vi "WS1050_Bench_RFFE_Package_FullStep_Multi-VPI_Ver1.4.vi"(4 "Send":bool, 5 "CLICK DOWN TO QUIT":bool=TRUE) -> (0 "EXE SEQ":bool, 1 "POWER ON":bool, 2 "CHARGE \nPUMP ON":bool, 3 "POWER OFF":bool)   [LabVIEW 2017]
uses:
  <instrlib>/Tektronix DPO MSO 2000 4000 Series/Tektronix DPO MSO 2000 4000 Series.lvlib
panel:
  in  "Driver Name":string[](array[string])=["C1_F1_UP", "C1_F1_DN", "C1_F2_UP", "C1_F2_DN", "C1_S1_UP", "C1_S2_UP", "C1_S3_UP", "C1_S4_UP", "C1_S5_UP", "C1_S6_UP", "C1_S7_UP", "C1_S8_UP", "C1_S9_UP", "C1_S10_UP", "C1_S11_UP", "C1_S12_UP", "C1_S13_UP", "C1_S14_UP", "C1_S13_DN", "C1_S12_DN", "C1_S11_DN", "C1_S10_DN", "C1_S9_DN", "C1_S8_DN", "C1_S7_DN", "C1_S6_DN", "C1_S5_DN", "C1_S4_DN", "C1_S3_DN", "C1_S2_DN", "C1_S1_DN", "C1_ALL_DN", "C2_F1_UP", "C2_F1_DN", "C2_F2_UP", "C2_F2_DN", "C2_S1_UP", "C2_S2_UP", "C2_S3_UP", "C2_S4_UP", "C2_S5_UP", "C2_S6_UP", "C2_S7_UP", "C2_S8_UP", "C2_S9_UP", "C2_S10_UP", "C2_S11_UP", "C2_S12_UP", "C2_S13_UP", "C2_S14_UP", "C2_S13_DN", "C2_S12_DN", "C2_S11_DN", "C2_S10_DN", "C2_S9_DN", "C2_S8_DN", "C2_S7_DN", "C2_S6_DN", "C2_S5_DN", "C2_S4_DN", "C2_S3_DN", "C2_S2_DN", "C2_S1_DN", "C2_ALL_DN", "C3_F1_UP", "C3_F1_DN", "C3_F2_UP", "C3_F2_DN", "C3_S1_UP", "C3_S2_UP", "C3_S3_UP", "C3_S4_UP", "C3_S5_UP", "C3_S6_UP", "C3_S7_UP", "C3_S8_UP", "C3_S9_UP", "C3_S10_UP", "C3_S11_UP", "C3_S12_UP", "C3_S13_UP", "C3_S14_UP", "C3_S13_DN", "C3_S12_DN", "C3_S11_DN", "C3_S10_DN", "C3_S9_DN", "C3_S8_DN", "C3_S7_DN", "C3_S6_DN", "C3_S5_DN", "C3_S4_DN", "C3_S3_DN", "C3_S2_DN", "C3_S1_DN", "C3_ALL_DN"]
  out "VPIData Out":string[][](array[string])=[["23.75", "24.688778E+0", "26.641948E+0", "1.143234E+0", "1.456892E+0", "1.305106E+0", "5.842594E+0", "6.189537E+0", "5.965014E+0", "1.144009E+0", "1.457367E+0", "1.305342E+0"], ["25.25", "28.907904E+0", "30.923880E+0", "1.143611E+0", "1.456986E+0", "1.305152E+0", "6.241702E+0", "6.610390E+0", "6.345839E+0", "1.144181E+0", "1.457457E+0", "1.305251E+0"], ["26.75", "29.144374E+0", "31.764876E+0", "1.143694E+0", "1.457180E+0", "1.305124E+0", "6.702805E+0", "7.218784E+0", "6.834179E+0", "1.144211E+0", "1.457512E+0", "1.305239E+0"], ["28.25", "34.886023E+0", "34.072784E+0", "1.143698E+0", "1.457273E+0", "1.305144E+0", "7.038370E+0", "7.580288E+0", "7.141688E+0", "1.144281E+0", "1.457594E+0", "1.305200E+0"], ["29.75", "39.362117E+0", "39.077158E+0", "1.143966E+0", "1.457275E+0", "1.304983E+0", "7.242981E+0", "7.704995E+0", "7.339693E+0", "1.144341E+0", "1.457691E+0", "1.305103E+0"], ["31.25", "42.309906E+0", "40.849836E+0", "1.143915E+0", "1.457288E+0", "1.304925E+0", "7.277188E+0", "7.740502E+0", "7.479733E+0", "1.144306E+0", "1.457570E+0", "1.305177E+0"], ["32.75", "44.234610E+0", "46.055910E+0", "1.143960E+0", "1.457368E+0", "1.305002E+0", "7.280773E+0", "7.734846E+0", "7.488937E+0", "1.144393E+0", "1.457617E+0", "1.305036E+0"], ["36.5", "53.659837E+0", "54.632880E+0", "1.143940E+0", "1.457204E+0", "1.304867E+0", "7.259427E+0", "7.702645E+0", "7.475886E+0", "1.144397E+0", "1.457589E+0", "1.304969E+0"], ["38", "59.644864E+0", "60.152367E+0", "1.143951E+0", "1.457364E+0", "1.304848E+0", "7.261446E+0", "7.706233E+0", "7.483841E+0", "1.144378E+0", "1.457810E+0", "1.304931E+0"], ["39.5", "63.989183E+0", "65.317284E+0", "1.143941E+0", "1.457225E+0", "1.304758E+0", "7.265702E+0", "7.716856E+0", "7.496982E+0", "1.144459E+0", "1.457567E+0", "1.305018E+0"], ["41", "71.621806E+0", "72.420343E+0", "1.143974E+0", "1.457385E+0", "1.304771E+0", "7.280796E+0", "7.729684E+0", "7.509736E+0", "1.144398E+0", "1.457685E+0", "1.304964E+0"], ["42.5", "79.427320E+0", "78.815208E+0", "1.144006E+0", "1.457337E+0", "1.304647E+0", "7.294107E+0", "7.742713E+0", "7.524602E+0", "1.144470E+0", "1.457591E+0", "1.304984E+0"], ["50", "124.732767E+0", "124.448999E+0", "1.143917E+0", "1.457358E+0", "1.304779E+0", "7.355203E+0", "7.811398E+0", "7.595755E+0", "1.144361E+0", "1.457583E+0", "1.304904E+0"]]
  in  "Sequence Names_Test":string[](array[string])=["CMin_VPI", "C1_VPI", "C2_VPI", "C3_VPI", "ALL_ON_VPI", "ALL_OFF_VPI"]
  out "Bank C1":string[](array[string])=["1.263962E+0", "1.365449E+0", "1.485278E+0", "1.432169E+0", "1.551803E+0", "1.653654E+0", "1.773449E+0", "1.874928E+0", "1.994661E+0", "2.096378E+0", "2.216085E+0", "2.295742E+0", "2.415533E+0", "2.517390E+0", "2.637083E+0", "2.682913E+0", "2.802580E+0", "2.904045E+0", "3.023833E+0", "3.131829E+0", "3.251440E+0", "3.353096E+0", "3.472585E+0", "3.523851E+0", "3.643284E+0", "3.745093E+0", "3.864497E+0", "3.961956E+0", "4.081577E+0", "4.183076E+0", "4.302464E+0", "4.402392E+0", "4.521881E+0", "4.623312E+0", "4.742844E+0", "4.829751E+0", "4.949292E+0", "5.050642E+0", "5.170100E+0", "5.220759E+0", "5.340368E+0", "5.441944E+0", "5.561578E+0", "5.635534E+0", "5.754912E+0", "5.856368E+0", "5.975750E+0", "6.045793E+0", "6.165061E+0", "6.266516E+0", "6.385998E+0", "6.487936E+0", "6.607210E+0", "6.708605E+0", "6.827699E+0", "6.897334E+0", "7.016852E+0", "7.117872E+0", "7.237418E+0", "7.119044E+0", "7.017414E+0", "6.898357E+0", "6.828583E+0", "6.709397E+0", "6.608499E+0", "6.489420E+0", "6.387433E+0", "6.268261E+0", "6.167466E+0", "6.048157E+0", "5.978147E+0", "5.859144E+0", "5.757853E+0", "5.638742E+0", "5.564712E+0", "5.445596E+0", "5.344232E+0", "5.225011E+0", "5.172354E+0", "5.053104E+0", "4.951765E+0", "4.832427E+0", "4.745420E+0", "4.626077E+0", "4.524684E+0", "4.405379E+0", "4.305223E+0", "4.185939E+0", "4.084376E+0", "3.964977E+0", "3.867230E+0", "3.747748E+0", "3.646212E+0", "3.526797E+0", "3.475012E+0", "3.355543E+0", "3.253861E+0", "3.134287E+0", "3.026013E+0", "2.906604E+0", "2.804812E+0", "2.685213E+0", "2.639527E+0", "2.519887E+0", "2.418143E+0", "2.298505E+0", "2.217875E+0", "2.098228E+0", "1.996638E+0", "1.876815E+0", "1.775184E+0", "1.655537E+0", "1.553577E+0", "1.433939E+0", "1.486023E+0", "1.366138E+0", "1.264338E+0", "1.144571E+0"]
  in  "Cmd Full":string[](array[string])=["01", "02", "03", "04", "05", "06", "07", "08", "09", "0A", "0B", "0C", "0D", "0E", "0F", "10", "11", "12", "13", "14", "15", "16", "17", "18", "19", "1A", "1B", "1C", "1D", "1E", "1F", "20", "21", "22", "23", "24", "25", "26", "27", "28", "29", "2A", "2B", "2C", "2D", "2E", "2F", "30", "31", "32", "33", "34", "35", "36", "37", "38", "39", "3A", "3B", "3A", "39", "38", "37", "36", "35", "34", "33", "32", "31", "30", "2F", "2E", "2D", "2C", "2B", "2A", "29", "28", "27", "26", "25", "24", "23", "22", "21", "20", "1F", "1E", "1D", "1C", "1B", "1A", "19", "18", "17", "16", "15", "14", "13", "12", "11", "10", "0F", "0E", "0D", "0C", "0B", "0A", "09", "08", "07", "06", "05", "04", "03", "02", "01", "00"]
  in  "Driver Name Full":string[](array[string])=["S0F1_UP", "S0F2_UP", "S0F12_UP", "S1_UP", "S1F1_UP", "S1F2_UP", "S1F12_UP", "S2_UP", "S2F1_UP", "S2F2_UP", "S2F12_UP", "S3_UP", "S3F1_UP", "S3F2_UP", "S3F12_UP", "S4_UP", "S4F1_UP", "S4F2_UP", "S4F12_UP", "S5_UP", "S5F1_UP", "S5F2_UP", "S5F12_UP", "S6_UP", "S6F1_UP", "S6F2_UP", "S6F12_UP", "S7_UP", "S7F1_UP", "S7F2_UP", "S7F12_UP", "S8_UP", "S8F1_UP", "S8F2_UP", "S8F12_UP", "S9_UP", "S9F1_UP", "S9F2_UP", "S9F12_UP", "S10_UP", "S10F1_UP", "S10F2_UP", "S10F12_UP", "S11_UP", "S11F1_UP", "S11F2_UP", "S11F12_UP", "S12_UP", "S12F1_UP", "S12F2_UP", "S12F12_UP", "S13_UP", "S13F1_UP", "S13F2_UP", "S13F12_UP", "S14_UP", "S14F1_UP", "S14F2_UP", "S14F12_UP", "S14F2_DN", "S14F1_DN", "S14_DN", "S13F12_DN", "S13F2_DN", "S13F1_DN", "S13_DN", "S12F12_DN", "S12F2_DN", "S12F1_DN", "S12_DN", "S11F12_DN", "S11F2_DN", "S11F1_DN", "S11_DN", "S10F12_DN", "S10F2_DN", "S10F1_DN", "S10_DN", "S9F12_DN", "S9F2_DN", "S9F1_DN", "S9_DN", "S8F12_DN", "S8F2_DN", "S8F1_DN", "S8_DN", "S7F12_DN", "S7F2_DN", "S7F1_DN", "S7_DN", "S6F12_DN", "S6F2_DN", "S6F1_DN", "S6_DN", "S5F12_DN", "S5F2_DN", "S5F1_DN", "S5_DN", "S4F12_DN", "S4F2_DN", "S4F1_DN", "S4_DN", "S3F12_DN", "S3F2_DN", "S3F1_DN", "S3_DN", "S2F12_DN", "S2F2_DN", "S2F1_DN", "S2_DN", "S1F12_DN", "S1F2_DN", "S1F1_DN", "S1_DN", "S0F12_DN", "S0F2_DN", "S0F1_DN", "ALL_OFF"]
  in  "WS1050 C3L Cmd":string[](array[string])=["074301", "074300", "074302", "074300", "074304", "074308", "07430C", "074310", "074314", "074318", "07431C", "074320", "074324", "074328", "07432C", "074330", "074334", "074338", "074339", "07433B", "074339", "074338", "074334", "074330", "07432C", "074328", "074324", "074320", "07431C", "074318", "074314", "074310", "07430C", "074308", "074304", "074300"]
  in  "C3L":string[](array[string])=["C3L_S0F1_ON", "C3L_S0F1_OFF", "C3L_S0F2_ON", "C3L_S0F2_OFF", "C3L_S1_UP", "C3L_S2_UP", "C3L_S3_UP", "C3L_S4_UP", "C3L_S5_UP", "C3L_S6_UP", "C3L_S7_UP", "C3L_S8_UP", "C3L_S9_UP", "C3L_S10_UP", "C3L_S11_UP", "C3L_S12_UP", "C3L_S13_UP", "C3L_S14_UP", "C3L_S14F1_UP", "C3L_S14F12_UP", "C3L_S14F1_DN", "C3L_S14_DN", "C3L_S13_DN", "C3L_S12_DN", "C3L_S11_DN", "C3L_S10_DN", "C3L_S9_DN", "C3L_S8_DN", "C3L_S7_DN", "C3L_S6_DN", "C3L_S5_DN", "C3L_S4_DN", "C3L_S3_DN", "C3L_S2_DN", "C3L_S1_DN", "C3L_ALL_OFF"]
  in  "WS1050 C2L Cmd":string[](array[string])=["074201", "074200", "074202", "074200", "074204", "074208", "07420C", "074210", "074214", "074218", "07421C", "074220", "074224", "074228", "07422C", "074230", "074234", "074238", "074239", "07423B", "074239", "074238", "074234", "074230", "07422C", "074228", "074224", "074220", "07421C", "074218", "074214", "074210", "07420C", "074208", "074204", "074200"]
  in  "C2L":string[](array[string])=["C2L_S0F1_ON", "C2L_S0F1_OFF", "C2L_S0F2_ON", "C2L_S0F2_OFF", "C2L_S1_UP", "C2L_S2_UP", "C2L_S3_UP", "C2L_S4_UP", "C2L_S5_UP", "C2L_S6_UP", "C2L_S7_UP", "C2L_S8_UP", "C2L_S9_UP", "C2L_S10_UP", "C2L_S11_UP", "C2L_S12_UP", "C2L_S13_UP", "C2L_S14_UP", "C2L_S14F1_UP", "C2L_S14F12_UP", "C2L_S14F1_DN", "C2L_S14_DN", "C2L_S13_DN", "C2L_S12_DN", "C2L_S11_DN", "C2L_S10_DN", "C2L_S9_DN", "C2L_S8_DN", "C2L_S7_DN", "C2L_S6_DN", "C2L_S5_DN", "C2L_S4_DN", "C2L_S3_DN", "C2L_S2_DN", "C2L_S1_DN", "C2L_ALL_OFF"]
  in  "C1 Cmd":string[](array[string])=["074101", "074100", "074102", "074100", "074104", "074108", "07410C", "074110", "074114", "074118", "07411C", "074120", "074124", "074128", "07412C", "074130", "074134", "074138", "074139", "07413B", "074139", "074138", "074134", "074130", "07412C", "074128", "074124", "074120", "07411C", "074118", "074114", "074110", "07410C", "074108", "074104", "074100"]
  in  "C1":string[](array[string])=["C1L_S0F1_ON", "C1L_S0F1_OFF", "C1L_S0F2_ON", "C1L_S0F2_OFF", "C1L_S1_UP", "C1L_S2_UP", "C1L_S3_UP", "C1L_S4_UP", "C1L_S5_UP", "C1L_S6_UP", "C1L_S7_UP", "C1L_S8_UP", "C1L_S9_UP", "C1L_S10_UP", "C1L_S11_UP", "C1L_S12_UP", "C1L_S13_UP", "C1L_S14_UP", "C1L_S14F1_UP", "C1L_S14F12_UP", "C1L_S14F1_DN", "C1L_S14_DN", "C1L_S13_DN", "C1L_S12_DN", "C1L_S11_DN", "C1L_S10_DN", "C1L_S9_DN", "C1L_S8_DN", "C1L_S7_DN", "C1L_S6_DN", "C1L_S5_DN", "C1L_S4_DN", "C1L_S3_DN", "C1L_S2_DN", "C1L_S1_DN", "C1L_ALL_OFF"]
  out "CMin Delay_AST":string[](array[string])=["0.000000E+0", "1.143716E+0", "1.458036E+0", "1.306985E+0", "0.000000E+0", "1.143733E+0", "1.457970E+0", "1.306825E+0", "0.000000E+0", "1.143759E+0", "1.458098E+0", "1.306746E+0", "0.000000E+0", "1.143710E+0", "1.457896E+0", "1.306740E+0"]
  in  "Reg1_Bit Cntrl 2":string[](array[string])=["01", "02", "04", "08", "10", "20", "40", "80", "03", "06", "0C", "D8", "33", "66", "CC", "07", "0E", "1C", "38", "70", "E0", "0F", "1E", "3C", "78", "F0", "1F", "3E", "7C", "F8", "3F", "7E", "FC", "7F", "FE", "FD", "FB", "F7", "EF", "DF", "BF", "7F", "FC", "F9", "F3", "E7", "CF", "9F", "3F", "F8", "F1", "E3", "C7", "8F", "1F", "F0", "E1", "C3", "87", "0F", "E0", "C1", "83", "07", "C0", "81", "03", "AA", "55", "00"]
  out "CMin C3(pF)":dbl=1.3051738281250005
  out "Delta_C3(pF)":dbl=6.016130171874999
  out "CMin C2(pF)":dbl=1.4578437500000003
  out "Delta_C2(pF)":dbl=6.2455592499999995
  out "Delta_C1(pF)":dbl=6.0930322578125
  out "CMin C1(pF)":dbl=1.1443857421874997
  in  "Tab Control":T1(tab)=enum."Indicator"
  in  "Select CPV":i32(ring)=1 items=["CP_35V", "CP_40.25V", "CP_41V", "CP_42.5V", "CP_44V", "CP_50V", "CP_55V"]
  in  "Header Table":string[][](table)=[["Lot#", "Wafer#", "SN#", "", "", "", "", "", "I_total"], ["WS1050", "T7", "1", "", "", "", "", "", "0.000000E+0"]]
  in  "TMN DC\\CAP Data Log File Path":path=path "C:/Andy/WS1050/Full TP/Multi VPI"
  out "2K Cycles":bool
  out "Pass /Fail?":bool=TRUE
  in  "Config File Path":path=path "S:/Software_Control/RELEASED_SOFTWARE_RUN_ALL_TEST_FROM_HERE/PACKAGE/TMN/TMN1P5-Test-System/WS1050_vsa20-20_Temp.txt"
  in  "Title":string="WS1050_Bench_RFFE_Package_Full_Multi-VPI Ver1.4"
  in  "Allowed (pF)":dbl=1.9898
  out "Difference":dbl=0.04109082031250022
  out "IDD_Stdby":string="652.477375E-3"
  out "C2Cal (pF)":dbl=-4.9191376953125
  out "C1Cal (pF)":dbl=-4.5642919921875
  out "C3Cal (pF)":dbl=-4.9974111328125
  in  "Bench #":string="1A"
  in  "Init AD7747":bool
  out "% Delta Cap":dbl=82.95919403248587 format="%#_5g"
  in  "VDD \nSet Up":dbl=3.3 format="%.2p"
  out "C2":dbl=1.4562451171874997
  out "C3":dbl=1.3041181640625004
  out "C1":dbl=1.1432705078124998
  in  "S-Time":bool=TRUE
  in  "GROUP":string
  out "HS \nCheck":bool=TRUE
  in  "Delay Cap Meas":u32=100
  out "Sequence":i32(listbox)=5
  out "IDD_All ON":string="36.261307E+0"
  out "IDD_All OFF":string="34.905880E+0"
  in  "Scope Set Up":bool
  in  "Manual CP Setting":i32(ring) items=["CP OFF", "CP ON", "DVA OFF", "DVA ON", "ECAL OFF", "ECAL ON", "CP 40.25V", "CP 35V", "CP 38V", "CP 44V", "CP 50V", "CP 23.75V", "CP 25.25V", "CP 29.75V", "C1 ON", "C1 OFF", "C2 ON", "C2 OFF", "C3 ON", "C3 OFF"]
  out "Bins":string="111111111"
  in  "Calib\nSocket":bool
  in  "BurnIn Efuse":bool
  out "S_ValueC2(pF)":dbl=-4.9191376953125
  out "S_ValueC1(pF)":dbl=-4.5642919921875
  out "S_ValueC3(pF)":dbl=-4.9974111328125
  out "Status":string="Idle....."
  in  "CMOS Setup":T2={"ECAL"=FALSE, "Full Steps"=TRUE, "Multi VPI"=TRUE, "DVA"=FALSE, "EFuse RB"=TRUE, "Init RB"=TRUE, "HS Test"=TRUE}
  in  "Comment":string="Init Run"
  out "IDD_VPI ON":string="124.448999E+0"
  out "IDD_VPI OFF":string="43.360206E+0"
  in  "Delta C Target":dbl=22.125
  in  "IDD Limit":dbl=0.02 format="%.2p"
  out "CMOS Out":T3
  out "Pass/Fail":bool
  in  "START \nTEST":bool
  in  "Save/Recal":u16(ring)=1 items=["Save", "Recall"]
  in  "Location":u16(ring)=1 items=["Location 1"=1, "Location 2"=2, "Location 3"=3, "Location 4"=4, "Location 5"=5, "Location 6"=6, "Location 7"=7, "Location 8"=8, "Location 9"=9, "Location 10"=10]
  in  "Dev 6501":tag="Dev2/port2/line0" caption="Lines"
  in  "Ke2400_VSA":refnum<visa-resource-name>="GPIB1::1::INSTR"
  in  "Scope USB":refnum<visa-resource-name>="USB0::0x0699::0x0405::C010240::INSTR"
  in  "Ke2000_IDD":refnum<visa-resource-name>="GPIB1::9::INSTR"
  in  "A364X_VDD":refnum<visa-resource-name>="GPIB1::6::INSTR"
  in  "RFFE":refnum<visa-resource-name>="COM3"
  in  "CAP Meas":refnum<visa-resource-name>="COM8"
  in  "% Amp_T2":dbl=0.9
  in  "% Amp_T1":dbl=0.6
  in  "% Amp_T3":dbl=0.95
  out "C1 Graph":dbl[](graph)=[0.0, 1.263962, 1.365449, 1.485278, 1.432169, 1.551803, 1.653654, 1.773449, 1.874928, 1.994661, 2.096378, 2.216085, 2.295742, 2.415533, 2.51739, 2.637083, 2.682913, 2.80258, 2.904045, 3.023833, 3.131829, 3.25144, 3.353096, 3.472585, 3.523851, 3.643284, 3.745093, 3.864497, 3.961956, 4.081577, 4.183076, 4.302464, 4.402392, 4.521881, 4.623312, 4.742844, 4.829751, 4.949292, 5.050642, 5.1701, 5.220759, 5.340368, 5.441944, 5.561578, 5.635534, 5.754912, 5.856368, 5.97575, 6.045793, 6.165061, 6.266516, 6.385998, 6.487936, 6.60721, 6.708605, 6.827699, 6.897334, 7.016852, 7.117872, 7.237418, 7.119044, 7.017414, 6.898357, 6.828583, 6.709397, 6.608499, 6.48942, 6.387433, 6.268261, 6.167466, 6.048157, 5.978147, 5.859144, 5.757853, 5.638742, 5.564712, 5.445596, 5.344232, 5.225011, 5.172354, 5.053104, 4.951765, 4.832427, 4.74542, 4.626077, 4.524684, 4.405379, 4.305223, 4.185939, 4.084376, 3.964977, 3.86723, 3.747748, 3.646212, 3.526797, 3.475012, 3.355543, 3.253861, 3.134287, 3.026013, 2.906604, 2.804812, 2.685213, 2.639527, 2.519887, 2.418143, 2.298505, 2.217875, 2.098228, 1.996638, 1.876815, 1.775184, 1.655537, 1.553577, 1.433939, 1.486023, 1.366138, 1.264338, 1.144571]
  out "C3 Graph":dbl[](graph)=[0.0, 1.422279, 1.529396, 1.647592, 1.587427, 1.705936, 1.813056, 1.931501, 2.010594, 2.12888, 2.236136, 2.354354, 2.442663, 2.560794, 2.668117, 2.786146, 2.836266, 2.954609, 3.061958, 3.180341, 3.261733, 3.37968, 3.48677, 3.605037, 3.668454, 3.787129, 3.894527, 4.012835, 4.070176, 4.188148, 4.295722, 4.413869, 4.460793, 4.579203, 4.686998, 4.804826, 4.863056, 4.981473, 5.088459, 5.206437, 5.295951, 5.414221, 5.521045, 5.638942, 5.718083, 5.835798, 5.942316, 6.060159, 6.166447, 6.284119, 6.391635, 6.509771, 6.557677, 6.675995, 6.782858, 6.900237, 6.978327, 7.095955, 7.202923, 7.321304, 7.203739, 7.097227, 6.979802, 6.901916, 6.784847, 6.678636, 6.561449, 6.514128, 6.396538, 6.289368, 6.171697, 6.065714, 5.948443, 5.841961, 5.725111, 5.645481, 5.528093, 5.421427, 5.303914, 5.214352, 5.097081, 4.990326, 4.87318, 4.814867, 4.69695, 4.590414, 4.473239, 4.422443, 4.3051, 4.197548, 4.08006, 4.021558, 3.903968, 3.797943, 3.679766, 3.609854, 3.491904, 3.384882, 3.266992, 3.185201, 3.067382, 2.960379, 2.842307, 2.791841, 2.673946, 2.566588, 2.448998, 2.359516, 2.241886, 2.135073, 2.016561, 1.936616, 1.818586, 1.711329, 1.593368, 1.648649, 1.53052, 1.423407, 1.305246]
  out "C2 Graph":dbl[](graph)=[0.0, 1.585713, 1.689148, 1.817662, 1.885455, 2.014188, 2.117619, 2.24629, 2.237105, 2.36588, 2.469066, 2.597716, 2.654179, 2.782699, 2.886215, 3.01476, 3.089162, 3.217774, 3.321294, 3.449749, 3.491522, 3.620192, 3.723275, 3.851945, 3.887914, 4.016458, 4.119716, 4.248221, 4.339437, 4.467828, 4.570915, 4.6994, 4.71226, 4.840867, 4.944326, 5.072629, 5.17246, 5.301332, 5.404473, 5.532792, 5.631586, 5.759431, 5.862757, 5.990751, 6.053234, 6.181604, 6.284377, 6.412689, 6.511694, 6.639869, 6.743027, 6.87107, 6.936174, 7.064378, 7.167445, 7.295804, 7.344181, 7.472198, 7.575125, 7.703403, 7.57569, 7.472819, 7.345312, 7.296507, 7.168775, 7.06663, 6.93829, 6.872623, 6.744731, 6.642141, 6.513973, 6.41498, 6.28691, 6.183715, 6.055874, 5.993849, 5.86599, 5.762587, 5.63454, 5.535872, 5.407794, 5.304726, 5.176538, 5.076043, 4.947812, 4.845088, 4.716747, 4.702071, 4.573709, 4.470539, 4.342157, 4.250793, 4.122445, 4.019188, 3.890785, 3.854401, 3.725925, 3.622958, 3.494537, 3.452021, 3.323469, 3.220432, 3.091716, 3.016233, 2.887631, 2.784359, 2.655705, 2.598903, 2.470368, 2.36705, 2.23842, 2.247739, 2.119168, 2.01572, 1.887002, 1.81881, 1.690278, 1.586776, 1.45797]
  out "Init EFuse RB":string[](array[string])=["40", "00", "00", "00", "28", "50", "00", "F3", "00", "00"]
  out "EFuse 1":string="50"
  out "EFuse 2":string="50"
  out "EUSE Burn":string[](array[string])=["n/a", "n/a"]
  out "I_stdby End":string="99.571387E+0"
  out "RB All Regs Dump":string[](array[string])=["44", "3B", "3B", "3B", "28", "50", "00", "F3", "00", "00", "44", "00", "00", "00", "28", "50", "00", "F3", "00", "00", "44", "00", "00", "00", "28", "50", "00", "EF", "20", "00", "44", "3B", "3B", "3B", "28", "50", "00", "EF", "20", "00", "44", "00", "00", "00", "28", "50", "00", "FB", "20", "00", "44", "3B", "3B", "3B", "28", "50", "00", "FB", "20", "00", "44", "00", "00", "00", "28", "50", "00", "F6", "20", "00", "44", "3B", "3B", "3B", "28", "50", "00", "F6", "20", "00"]
  in  "RB All Regs":bool=TRUE
  in  "CMin Delay":string[](array[string])=["0", "0", "0", "0"]
  in  "CMin/Delay":bool
  out "Ke2400 out":refnum<visa-resource-name>
  out "VDD Out Dup":refnum<visa-resource-name>
  out "Error Out":errorcluster
  out "AST":errorcluster
  out "Completed":errorcluster
  out "RFFE Out After Test":errorcluster
  out "Signal":dbl[](graph)
  out "Filtered Signal":dbl[](graph)
  out "After RB":errorcluster
  out "Power OFF":errorcluster
  out "Lot":string="WS1050"
  out "Wafer":string="T7"
  out "All Out":string[](array[string])=["4/7/2014", "4:26:21 PM", "WS1050", "T7", "1", "40", "00", "00", "00", "28", "50", "00", "F3", "00", "00", "Pass", "50", "50", "652.477375E-3", "34.905880E+0", "36.261307E+0", "1.144386E+0", "1.457844E+0", "1.305174E+0", "1.263962E+0", "1.365449E+0", "1.485278E+0", "1.432169E+0", "1.551803E+0", "1.653654E+0", "1.773449E+0", "1.874928E+0", "1.994661E+0", "2.096378E+0", "2.216085E+0", "2.295742E+0", "2.415533E+0", "2.517390E+0", "2.637083E+0", "2.682913E+0", "2.802580E+0", "2.904045E+0", "3.023833E+0", "3.131829E+0", "3.251440E+0", "3.353096E+0", "3.472585E+0", "3.523851E+0", "3.643284E+0", "3.745093E+0", "3.864497E+0", "3.961956E+0", "4.081577E+0", "4.183076E+0", "4.302464E+0", "4.402392E+0", "4.521881E+0", "4.623312E+0", "4.742844E+0", "4.829751E+0", "4.949292E+0", "5.050642E+0", "5.170100E+0", "5.220759E+0", "5.340368E+0", "5.441944E+0", "5.561578E+0", "5.635534E+0", "5.754912E+0", "5.856368E+0", "5.975750E+0", "6.045793E+0", "6.165061E+0", "6.266516E+0", "6.385998E+0", "6.487936E+0", "6.607210E+0", "6.708605E+0", "6.827699E+0", "6.897334E+0", "7.016852E+0", "7.117872E+0", "7.237418E+0", "7.119044E+0", "7.017414E+0", "6.898357E+0", "6.828583E+0", "6.709397E+0", "6.608499E+0", "6.489420E+0", "6.387433E+0", "6.268261E+0", "6.167466E+0", "6.048157E+0", "5.978147E+0", "5.859144E+0", "5.757853E+0", "5.638742E+0", "5.564712E+0", "5.445596E+0", "5.344232E+0", "5.225011E+0", "5.172354E+0", "5.053104E+0", "4.951765E+0", "4.832427E+0", "4.745420E+0", "4.626077E+0", "4.524684E+0", "4.405379E+0", "4.305223E+0", "4.185939E+0", "4.084376E+0", "3.964977E+0", "3.867230E+0", "3.747748E+0", "3.646212E+0", "3.526797E+0", "3.475012E+0", "3.355543E+0", "3.253861E+0", "3.134287E+0", "3.026013E+0", "2.906604E+0", "2.804812E+0", "2.685213E+0", "2.639527E+0", "2.519887E+0", "2.418143E+0", "2.298505E+0", "2.217875E+0", "2.098228E+0", "1.996638E+0", "1.876815E+0", "1.775184E+0", "1.655537E+0", "1.553577E+0", "1.433939E+0", "1.486023E+0", "1.366138E+0", "1.264338E+0", "1.144571E+0", "1.195763E-1", "2.210633E-1", "3.408923E-1", "2.877833E-1", "4.074173E-1", "5.092683E-1", "6.290633E-1", "7.305423E-1", "8.502753E-1", "9.519923E-1", "1.071699E+0", "1.151356E+0", "1.271147E+0", "1.373004E+0", "1.492697E+0", "1.538527E+0", "1.658194E+0", "1.759659E+0", "1.879447E+0", "1.987443E+0", "2.107054E+0", "2.208710E+0", "2.328199E+0", "2.379465E+0", "2.498898E+0", "2.600707E+0", "2.720111E+0", "2.817570E+0", "2.937191E+0", "3.038690E+0", "3.158078E+0", "3.258006E+0", "3.377495E+0", "3.478926E+0", "3.598458E+0", "3.685365E+0", "3.804906E+0", "3.906256E+0", "4.025714E+0", "4.076373E+0", "4.195982E+0", "4.297558E+0", "4.417192E+0", "4.491148E+0", "4.610526E+0", "4.711982E+0", "4.831364E+0", "4.901407E+0", "5.020675E+0", "5.122130E+0", "5.241612E+0", "5.343550E+0", "5.462824E+0", "5.564219E+0", "5.683313E+0", "5.752948E+0", "5.872466E+0", "5.973486E+0", "3.760000E-4", "6.890000E-4", "7.450000E-4", "1.770000E-3", "1.774000E-3", "1.883000E-3", "1.735000E-3", "1.887000E-3", "1.977000E-3", "1.850000E-3", "1.790000E-3", "2.763000E-3", "2.610000E-3", "2.497000E-3", "2.444000E-3", "2.300000E-3", "2.232000E-3", "2.559000E-3", "2.180000E-3", "2.458000E-3", "2.421000E-3", "2.447000E-3", "2.427000E-3", "2.946000E-3", "2.928000E-3", "2.655000E-3", "2.733000E-3", "3.021000E-3", "2.799000E-3", "2.863000E-3", "2.759000E-3", "2.987000E-3", "2.803000E-3", "2.765000E-3", "2.576000E-3", "2.676000E-3", "2.473000E-3", "2.462000E-3", "2.254000E-3", "4.252000E-3", "3.864000E-3", "3.652000E-3", "3.134000E-3", "3.208000E-3", "2.941000E-3", "2.776000E-3", "2.397000E-3", "2.364000E-3", "2.405000E-3", "1.745000E-3", "1.435000E-3", "1.484000E-3", "1.289000E-3", "7.920000E-4", "8.840000E-4", "1.023000E-3", "5.620000E-4", "1.172000E-3", "1.585713E+0", "1.689148E+0", "1.817662E+0", "1.885455E+0", "2.014188E+0", "2.117619E+0", "2.246290E+0", "2.237105E+0", "2.365880E+0", "2.469066E+0", "2.597716E+0", "2.654179E+0", "2.782699E+0", "2.886215E+0", "3.014760E+0", "3.089162E+0", "3.217774E+0", "3.321294E+0", "3.449749E+0", "3.491522E+0", "3.620192E+0", "3.723275E+0", "3.851945E+0", "3.887914E+0", "4.016458E+0", "4.119716E+0", "4.248221E+0", "4.339437E+0", "4.467828E+0", "4.570915E+0", "4.699400E+0", "4.712260E+0", "4.840867E+0", "4.944326E+0", "5.072629E+0", "5.172460E+0", "5.301332E+0", "5.404473E+0", "5.532792E+0", "5.631586E+0", "5.759431E+0", "5.862757E+0", "5.990751E+0", "6.053234E+0", "6.181604E+0", "6.284377E+0", "6.412689E+0", "6.511694E+0", "6.639869E+0", "6.743027E+0", "6.871070E+0", "6.936174E+0", "7.064378E+0", "7.167445E+0", "7.295804E+0", "7.344181E+0", "7.472198E+0", "7.575125E+0", "7.703403E+0", "7.575690E+0", "7.472819E+0", "7.345312E+0", "7.296507E+0", "7.168775E+0", "7.066630E+0", "6.938290E+0", "6.872623E+0", "6.744731E+0", "6.642141E+0", "6.513973E+0", "6.414980E+0", "6.286910E+0", "6.183715E+0", "6.055874E+0", "5.993849E+0", "5.865990E+0", "5.762587E+0", "5.634540E+0", "5.535872E+0", "5.407794E+0", "5.304726E+0", "5.176538E+0", "5.076043E+0", "4.947812E+0", "4.845088E+0", "4.716747E+0", "4.702071E+0", "4.573709E+0", "4.470539E+0", "4.342157E+0", "4.250793E+0", "4.122445E+0", "4.019188E+0", "3.890785E+0", "3.854401E+0", "3.725925E+0", "3.622958E+0", "3.494537E+0", "3.452021E+0", "3.323469E+0", "3.220432E+0", "3.091716E+0", "3.016233E+0", "2.887631E+0", "2.784359E+0", "2.655705E+0", "2.598903E+0", "2.470368E+0", "2.367050E+0", "2.238420E+0", "2.247739E+0", "2.119168E+0", "2.015720E+0", "1.887002E+0", "1.818810E+0", "1.690278E+0", "1.586776E+0", "1.457970E+0", "1.278692E-1", "2.313042E-1", "3.598182E-1", "4.276112E-1", "5.563442E-1", "6.597752E-1", "7.884462E-1", "7.792612E-1", "9.080362E-1", "1.011222E+0", "1.139872E+0", "1.196335E+0", "1.324855E+0", "1.428371E+0", "1.556916E+0", "1.631318E+0", "1.759930E+0", "1.863450E+0", "1.991905E+0", "2.033678E+0", "2.162348E+0", "2.265431E+0", "2.394101E+0", "2.430070E+0", "2.558614E+0", "2.661872E+0", "2.790377E+0", "2.881593E+0", "3.009984E+0", "3.113071E+0", "3.241556E+0", "3.254416E+0", "3.383023E+0", "3.486482E+0", "3.614785E+0", "3.714616E+0", "3.843488E+0", "3.946629E+0", "4.074948E+0", "4.173742E+0", "4.301587E+0", "4.404913E+0", "4.532907E+0", "4.595390E+0", "4.723760E+0", "4.826533E+0", "4.954845E+0", "5.053850E+0", "5.182025E+0", "5.285183E+0", "5.413226E+0", "5.478330E+0", "5.606534E+0", "5.709601E+0", "5.837960E+0", "5.886337E+0", "6.014354E+0", "6.117281E+0", "1.063000E-3", "1.130000E-3", "1.148000E-3", "1.547000E-3", "1.532000E-3", "1.549000E-3", "1.449000E-3", "1.315000E-3", "1.170000E-3", "1.302000E-3", "1.187000E-3", "1.526000E-3", "1.660000E-3", "1.416000E-3", "1.473000E-3", "2.554000E-3", "2.658000E-3", "2.175000E-3", "2.272000E-3", "3.015000E-3", "2.766000E-3", "2.650000E-3", "2.456000E-3", "2.871000E-3", "2.730000E-3", "2.729000E-3", "2.572000E-3", "2.720000E-3", "2.711000E-3", "2.794000E-3", "2.671000E-3", "4.487000E-3", "4.221000E-3", "3.486000E-3", "3.414000E-3", "4.078000E-3", "3.394000E-3", "3.321000E-3", "3.080000E-3", "2.954000E-3", "3.156000E-3", "3.233000E-3", "3.098000E-3", "2.640000E-3", "2.111000E-3", "2.533000E-3", "2.291000E-3", "2.279000E-3", "2.272000E-3", "1.704000E-3", "1.553000E-3", "2.116000E-3", "2.252000E-3", "1.330000E-3", "7.030000E-4", "1.131000E-3", "6.210000E-4", "5.650000E-4", "1.422279E+0", "1.529396E+0", "1.647592E+0", "1.587427E+0", "1.705936E+0", "1.813056E+0", "1.931501E+0", "2.010594E+0", "2.128880E+0", "2.236136E+0", "2.354354E+0", "2.442663E+0", "2.560794E+0", "2.668117E+0", "2.786146E+0", "2.836266E+0", "2.954609E+0", "3.061958E+0", "3.180341E+0", "3.261733E+0", "3.379680E+0", "3.486770E+0", "3.605037E+0", "3.668454E+0", "3.787129E+0", "3.894527E+0", "4.012835E+0", "4.070176E+0", "4.188148E+0", "4.295722E+0", "4.413869E+0", "4.460793E+0", "4.579203E+0", "4.686998E+0", "4.804826E+0", "4.863056E+0", "4.981473E+0", "5.088459E+0", "5.206437E+0", "5.295951E+0", "5.414221E+0", "5.521045E+0", "5.638942E+0", "5.718083E+0", "5.835798E+0", "5.942316E+0", "6.060159E+0", "6.166447E+0", "6.284119E+0", "6.391635E+0", "6.509771E+0", "6.557677E+0", "6.675995E+0", "6.782858E+0", "6.900237E+0", "6.978327E+0", "7.095955E+0", "7.202923E+0", "7.321304E+0", "7.203739E+0", "7.097227E+0", "6.979802E+0", "6.901916E+0", "6.784847E+0", "6.678636E+0", "6.561449E+0", "6.514128E+0", "6.396538E+0", "6.289368E+0", "6.171697E+0", "6.065714E+0", "5.948443E+0", "5.841961E+0", "5.725111E+0", "5.645481E+0", "5.528093E+0", "5.421427E+0", "5.303914E+0", "5.214352E+0", "5.097081E+0", "4.990326E+0", "4.873180E+0", "4.814867E+0", "4.696950E+0", "4.590414E+0", "4.473239E+0", "4.422443E+0", "4.305100E+0", "4.197548E+0", "4.080060E+0", "4.021558E+0", "3.903968E+0", "3.797943E+0", "3.679766E+0", "3.609854E+0", "3.491904E+0", "3.384882E+0", "3.266992E+0", "3.185201E+0", "3.067382E+0", "2.960379E+0", "2.842307E+0", "2.791841E+0", "2.673946E+0", "2.566588E+0", "2.448998E+0", "2.359516E+0", "2.241886E+0", "2.135073E+0", "2.016561E+0", "1.936616E+0", "1.818586E+0", "1.711329E+0", "1.593368E+0", "1.648649E+0", "1.530520E+0", "1.423407E+0", "1.305246E+0", "1.171052E-1", "2.242222E-1", "3.424182E-1", "2.822532E-1", "4.007622E-1", "5.078822E-1", "6.263272E-1", "7.054202E-1", "8.237062E-1", "9.309622E-1", "1.049180E+0", "1.137489E+0", "1.255620E+0", "1.362943E+0", "1.480972E+0", "1.531092E+0", "1.649435E+0", "1.756784E+0", "1.875167E+0", "1.956559E+0", "2.074506E+0", "2.181596E+0", "2.299863E+0", "2.363280E+0", "2.481955E+0", "2.589353E+0", "2.707661E+0", "2.765002E+0", "2.882974E+0", "2.990548E+0", "3.108695E+0", "3.155619E+0", "3.274029E+0", "3.381824E+0", "3.499652E+0", "3.557882E+0", "3.676299E+0", "3.783285E+0", "3.901263E+0", "3.990777E+0", "4.109047E+0", "4.215871E+0", "4.333768E+0", "4.412909E+0", "4.530624E+0", "4.637142E+0", "4.754985E+0", "4.861273E+0", "4.978945E+0", "5.086461E+0", "5.204597E+0", "5.252503E+0", "5.370821E+0", "5.477684E+0", "5.595063E+0", "5.673153E+0", "5.790781E+0", "5.897749E+0", "1.128000E-3", "1.124000E-3", "1.057000E-3", "5.941000E-3", "5.393000E-3", "5.530000E-3", "5.115000E-3", "5.967000E-3", "6.193000E-3", "5.750000E-3", "5.162000E-3", "6.335000E-3", "5.794000E-3", "5.829000E-3", "5.695000E-3", "6.041000E-3", "5.770000E-3", "5.424000E-3", "4.860000E-3", "5.259000E-3", "5.202000E-3", "5.134000E-3", "4.817000E-3", "1.131200E-2", "1.081400E-2", "9.441000E-3", "8.723000E-3", "9.884000E-3", "9.400000E-3", "9.378000E-3", "8.574000E-3", "1.244600E-2", "1.121100E-2", "9.952000E-3", "1.004100E-2", "1.012400E-2", "8.853000E-3", "8.622000E-3", "7.915000E-3", "7.963000E-3", "7.206000E-3", "7.048000E-3", "6.539000E-3", "7.028000E-3", "6.163000E-3", "6.127000E-3", "5.555000E-3", "5.250000E-3", "5.249000E-3", "4.903000E-3", "4.357000E-3", "3.772000E-3", "2.641000E-3", "1.989000E-3", "1.679000E-3", "1.475000E-3", "1.272000E-3", "8.160000E-4", "23.75", "24.688778E+0", "26.641948E+0", "1.143234E+0", "1.456892E+0", "1.305106E+0", "5.842594E+0", "6.189537E+0", "5.965014E+0", "1.144009E+0", "1.457367E+0", "1.305342E+0", "25.25", "28.907904E+0", "30.923880E+0", "1.143611E+0", "1.456986E+0", "1.305152E+0", "6.241702E+0", "6.610390E+0", "6.345839E+0", "1.144181E+0", "1.457457E+0", "1.305251E+0", "26.75", "29.144374E+0", "31.764876E+0", "1.143694E+0", "1.457180E+0", "1.305124E+0", "6.702805E+0", "7.218784E+0", "6.834179E+0", "1.144211E+0", "1.457512E+0", "1.305239E+0", "28.25", "34.886023E+0", "34.072784E+0", "1.143698E+0", "1.457273E+0", "1.305144E+0", "7.038370E+0", "7.580288E+0", "7.141688E+0", "1.144281E+0", "1.457594E+0", "1.305200E+0", "29.75", "39.362117E+0", "39.077158E+0", "1.143966E+0", "1.457275E+0", "1.304983E+0", "7.242981E+0", "7.704995E+0", "7.339693E+0", "1.144341E+0", "1.457691E+0", "1.305103E+0", "31.25", "42.309906E+0", "40.849836E+0", "1.143915E+0", "1.457288E+0", "1.304925E+0", "7.277188E+0", "7.740502E+0", "7.479733E+0", "1.144306E+0", "1.457570E+0", "1.305177E+0", "32.75", "44.234610E+0", "46.055910E+0", "1.143960E+0", "1.457368E+0", "1.305002E+0", "7.280773E+0", "7.734846E+0", "7.488937E+0", "1.144393E+0", "1.457617E+0", "1.305036E+0", "36.5", "53.659837E+0", "54.632880E+0", "1.143940E+0", "1.457204E+0", "1.304867E+0", "7.259427E+0", "7.702645E+0", "7.475886E+0", "1.144397E+0", "1.457589E+0", "1.304969E+0", "38", "59.644864E+0", "60.152367E+0", "1.143951E+0", "1.457364E+0", "1.304848E+0", "7.261446E+0", "7.706233E+0", "7.483841E+0", "1.144378E+0", "1.457810E+0", "1.304931E+0", "39.5", "63.989183E+0", "65.317284E+0", "1.143941E+0", "1.457225E+0", "1.304758E+0", "7.265702E+0", "7.716856E+0", "7.496982E+0", "1.144459E+0", "1.457567E+0", "1.305018E+0", "41", "71.621806E+0", "72.420343E+0", "1.143974E+0", "1.457385E+0", "1.304771E+0", "7.280796E+0", "7.729684E+0", "7.509736E+0", "1.144398E+0", "1.457685E+0", "1.304964E+0", "42.5", "79.427320E+0", "78.815208E+0", "1.144006E+0", "1.457337E+0", "1.304647E+0", "7.294107E+0", "7.742713E+0", "7.524602E+0", "1.144470E+0", "1.457591E+0", "1.304984E+0", "50", "124.732767E+0", "124.448999E+0", "1.143917E+0", "1.457358E+0", "1.304779E+0", "7.355203E+0", "7.811398E+0", "7.595755E+0", "1.144361E+0", "1.457583E+0", "1.304904E+0", "51.283140E+0", "51.442790E+0", "1.143863E+0", "1.457229E+0", "1.304684E+0", "7.260558E+0", "7.715813E+0", "7.478388E+0", "1.144738E+0", "1.457998E+0", "1.305351E+0", "84.675790E+0", "83.862669E+0", "7.306897E+0", "7.755671E+0", "7.539573E+0", "1.144926E+0", "1.458117E+0", "1.305444E+0", "68.096661E+0", "67.783581E+0", "7.273860E+0", "7.722597E+0", "7.504744E+0", "1.145042E+0", "1.458205E+0", "1.305488E+0", "-2.000000E+1", "1.220885E+0", "1.545516E+0", "1.379979E+0", "0.000000E+0", "1.144338E+0", "1.457525E+0", "1.304988E+0", "2.000000E+1", "1.214448E+0", "1.552379E+0", "1.388416E+0", "0.000000E+0", "1.143961E+0", "1.457421E+0", "1.304836E+0", "0.000000E+0", "1.143805E+0", "1.457186E+0", "1.304919E+0", "0.000000E+0", "1.144008E+0", "1.457104E+0", "1.304849E+0", "0.000000E+0", "1.143882E+0", "1.457153E+0", "1.304773E+0"]
  in  "Bank Cmd":string[](array[string])=["074100", "07413B", "07423B", "07433B", "07413B", "074100"]
  in  "Delta C % Setting":dbl[](array[numeric])=[0.0, 70.0, 72.5, 75.0, 77.5, 80.0, 82.5, 85.0, 87.5, 90.0, 92.5, 95.0, 97.5, 100.0, 102.5, 105.0]
  out "C3(pF)":dbl=-8.192 format="%#_4g"
  out "C1(pF)":dbl=-8.192 format="%#_4g"
  out "C2(pF)":dbl=-8.192 format="%#_4g"
  in  "error in":errorcluster
  # "Company:  WiSpry Inc\n198 Fairbanks Ste 198 Irvine\n\nCreated by:  Andy V Tran\nDate:  07/09/2015\nTest Program:  WS1050 Bench\nTP_Bench RFFE Full Multi-VPI Ver1.4\nLabVIEW 2012 Professional"
  # "Note For Update:  Ver 1.4 updated based on Ver 1.3\n\n1.  Extract data to calculate RT and FT based on \n     a.  % of Amp for T1\n     b.  % of Amp for T2\n     c.  % of Amp for T3\n2.  Set noise level for 5mV\n3.  Calculated RT and FT start from CLK 21th."
  # "Monitor Errors Output"
  # "Binning Criteria:\n\nBin 1 = Pass\nBin 5 = Idd Stdby > 20uA; \nBin 6, E = IDD ON/OFF\n40uA < IDD On/OFF < 100uA; \nBin 8 = RTZ > 50fF each bank;\nBin 7 = CMax\n5pF < C1, C2, C3 < 8.129pF \nBin B = CMin; \n1.1pF < C1, C2, C3 < 1.8pF\nBin C = Delta Change > 10%\nBin 9 = VSA > 10% each bank\nTarget Delta Cap:  \nC1 = 7.375pF; C2 = 7.375pF; \nC3 = 7.375pF"
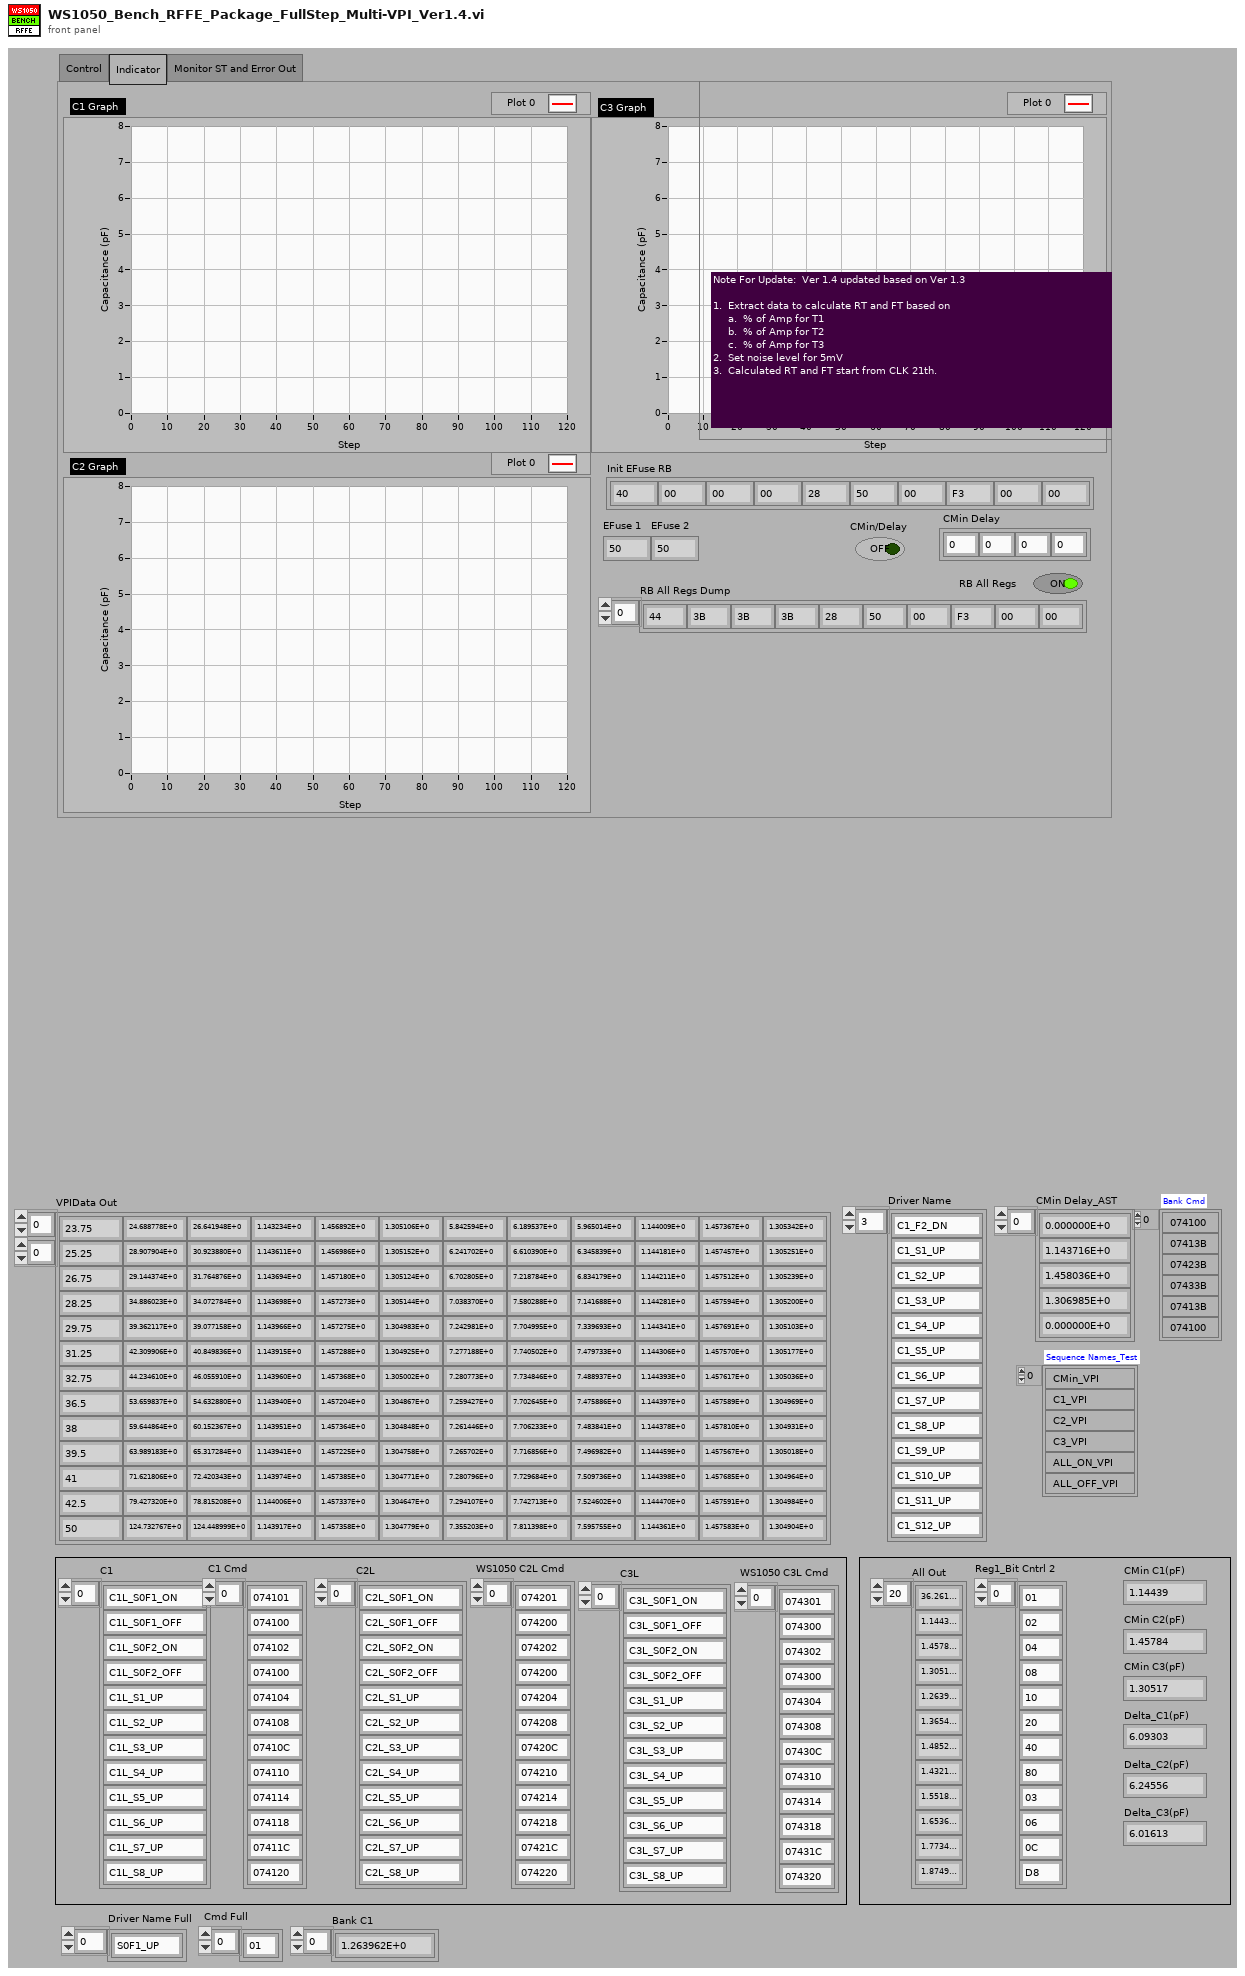
[diagram p1: front panel]
types:
  T1 = enum32{"Control", "Indicator", "Monitor ST and Error Out"}
  T2 = cluster{"ECAL":bool, "Full Steps":bool, "Multi VPI":bool, "DVA":bool, "EFuse RB":bool, "Init RB":bool, "HS Test":bool}
  T3 = cluster{"ECAL":bool, "DVA":bool, "Full Steps":bool, "Multi VPI":bool, "EFuse RB":bool, "Init RB":bool, "HS Test":bool}
  T4 = typedef "TSTR Configuration Cluster1.0.ctl" = cluster{"DeltaCA Low Limit ":dbl, "DeltaCA High Limit (V)":dbl, "DeltaCE Low Limit ":dbl, "DeltaCE High Limit":dbl, "DeltaCC Low Limit":dbl, "DeltaCC High Limit":dbl, "RTZ Limit":dbl, "Cmin Low Limit":dbl, "Cmin High Limit":dbl, "Idd High Limit (A)":dbl, "Idd Low Limit (A)":dbl, "Delta IDD":dbl, "Bin Path":string, "VSA Path1":string, "Dem Path":string, "Delay":dbl, "VSA":bool, "SWCyc":bool, "VPI":bool, "Bipolar":bool, "OVS Voltage":dbl, "Wait Time":dbl, "ATE":bool, "VNA GPIB":string, "Meter GPIB ":string, "Op level":string, "Idd Standby":dbl, "VSA Voltage1":dbl, "VSA Cap":dbl, "Test Name":string, "Nominal Trim Code":i32, "VPI Trim Code":i32, "De-Embd":bool, "Loop Count":i32, "Bipolar":bool, "VSA Path 2":string, "VSA Voltage2":dbl}
  T5 = cluster{"Bench #":string, "Title ":string, "Test Name":string, "Comment":string}
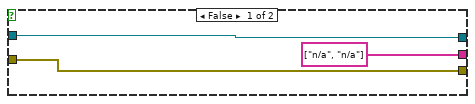
[diagram p5: hidden frame]
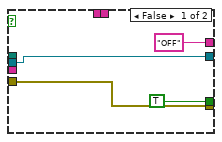
[diagram p6: hidden frame]
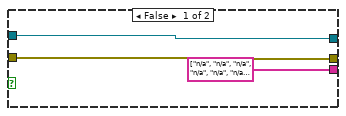
[diagram p7: hidden frame]
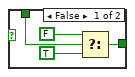
[diagram p9: hidden frame]
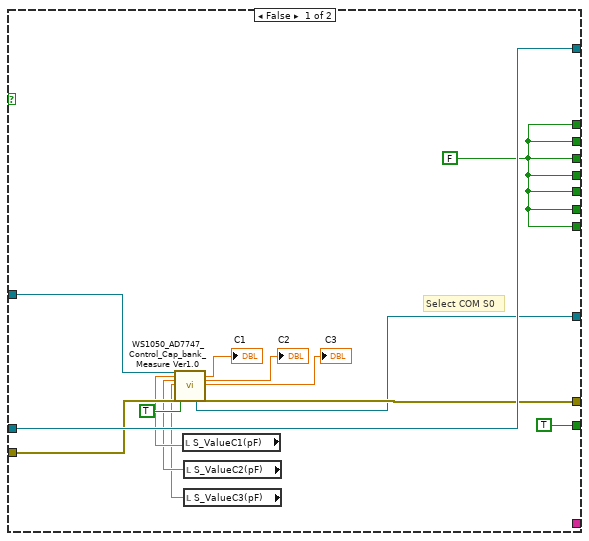
[diagram p13: hidden frame]
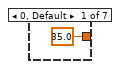
[diagram p14: hidden frame]
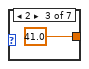
[diagram p15: hidden frame]
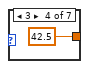
[diagram p16: hidden frame]
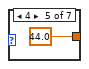
[diagram p17: hidden frame]
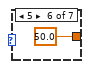
[diagram p18: hidden frame]
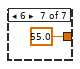
[diagram p19: hidden frame]
diagram:
  n1 = call "WS1050 Read From Configuration File.vi"("error in (no error)"="error in", "Configuration File Path"="Config File Path") -> ("error out"=w16:errorcluster, "Configuration"=w66:T4)  [unwired: 8 in]
  n2 = Format Into String(format string="%.;CURR %f", "IDD Limit") -> (resulting string=w39:string)  [unwired: 2 in, 1 out]
  n3 = VISA Open(error in (no error)=w16, VISA resource name="RFFE") -> (VISA resource name=w58:refnum<visa-resource-name>, error out=w57:errorcluster)  [unwired: 3 in]
  n4 = VISA Write(VISA resource name="A364X_VDD", write buffer="VOLT 0.0;:OUTP 1", error in (no error)=w16) -> (VISA resource name out=w38:refnum<visa-resource-name>, error out=w42:errorcluster)  [unwired: 1 out]
  n5 = call "Delay.vi"("error in (no error)"=w42, "milliseconds to wait"=u32 100) -> ("error out"=w37:errorcluster)  [unwired: 9 in]
  n6 = case shown="False" FALSE ("Relay_ 10") {
    tunnel: w16 -> [w72 w73]
    tunnel: [w69 w73] -> w14
    tunnel: "Dev 6501" -> [w68 _]
    frame False {
      w70 = FALSE ("Relay_ 10")
      w71 = u16 0 items=["All Off", "Bank 1", "Bank 2", "Bank 3"] ("Ring")
      n7 = call "WS105x_NI_6501_Relay_Control.vi"("Ring"=w71, "Lines"=w68, "Relay_ 11"=w70, "error in (no error)"=w72, "Relay_ 10"=w70) -> ("error out"=w69:errorcluster)  [unwired: 1 in, 9 out]
    }
    frame True {
    }
  }
  n8 = VISA Open(error in (no error)=w16, VISA resource name="CAP Meas") -> (VISA resource name=w62:refnum<visa-resource-name>, error out=w63:errorcluster)  [unwired: 3 in]
  n9 = case shown="True" TRUE {
    tunnel: "Scope USB" -> [w75 w80]
    tunnel: w16 -> [w74 w79]
    tunnel: [w75 w77] -> w18
    tunnel: [w74 w76] -> w17
    frame False {
    }
    frame True {
      w78 = TRUE ("ID Query")
      n10 = call <instrlib>:"Initialize.vi"("error in (no error)"=w79, "Reset (True)"=w78, "ID Query (True)"=w78, "VISA resource name"=w80) -> ("error out"=w76:errorcluster, "VISA resource name out"=w77:refnum<visa-resource-name>)  [unwired: 6 in]
    }
  }
  n11 = call "Ke2400 VI Controler.vi"("ON/OFF"=TRUE, "Voltage Range"=100 ("Voltage Range(V)"), "error in (no error)"=w16, "Current Compliace"=6.0 ("Current Compliance(mA)"), "Volt Level"=0.0 ("Volt Level(V)"), "VISA In"="Ke2400_VSA") -> ("error out"=w33:errorcluster, "VISA Out"=w34:refnum<visa-resource-name>)  [unwired: 4 in]
  n12 = call "Initialize_PIC.vi"("error in (no error)"=w57, "baud rate"=u32 9600, "Select Com Port"=w58) -> ("error out"=w56:errorcluster, "VISA resource name out"=w55:refnum<visa-resource-name>)  [unwired: 7 in]
  n13 = VISA Write(VISA resource name=w38, write buffer=w39, error in (no error)=w37) -> (VISA resource name out=w36:refnum<visa-resource-name>, error out=w35:errorcluster)  [unwired: 1 out]
  n14 = call "Initialize_PIC.vi"("error in (no error)"=w63, "baud rate"=u32 9600, "Select Com Port"=w62) -> ("error out"=w48:errorcluster, "VISA resource name out"=w54:refnum<visa-resource-name>)  [unwired: 7 in]
  n15 = VISA Write(VISA resource name=w55, write buffer="5", error in (no error)=w56) -> (VISA resource name out=w52:refnum<visa-resource-name>, error out=w53:errorcluster)  [unwired: 1 out]
  n16 = Merge Errors(w14, w48, w35, w33, w17) -> (w65:errorcluster)
  n17 = while {
    tunnel: w66 -> [w195]
    tunnel: "Config File Path" -> [w181]
    tunnel: [w193] -> w46
    tunnel: w66 -> [w184]
    tunnel: w54 -> [w115]
    tunnel: w34 -> [w173]
    tunnel: w36 -> [w84]
    tunnel: [w163] -> w11
    tunnel: [w162] -> w26
    tunnel: [w158] -> w25
    tunnel: w65 -> [w90]
    tunnel: [w157] -> w8
    tunnel: [w152] -> w12
    tunnel: "Ke2000_IDD" -> [w150]
    tunnel: [w126] -> w9
    tunnel: w53 -> [w89]
    tunnel: w52 -> [w87]
    tunnel: [w119] -> w7
    tunnel: w18 -> [w93]
    tunnel: [w82] -> w3
    i -> [w99]
    stop <- "CLICK DOWN TO QUIT" continue-if-true
    w132 = 1 ("index (row)")
    # "ECAL"
    # "DVA"
    # "Ke2400"
    # "2K"
    # "VDD"
    # "I2C"
    # "Multi VPI"
    n18 = case shown="True" "START \nTEST" {
      tunnel: [w391 w428] -> w141
      tunnel: [TRUE ("Pass/Fail") w435] -> w197
      tunnel: w115 -> [w390 w432]
      tunnel: w84 -> [w393 w414]
      tunnel: [w393 w408] -> w161
      tunnel: [w389 w429] -> w118
      tunnel: w90 -> [w392 w413]
      tunnel: [w381 w405] -> w145
      tunnel: [w381 w406] -> w125
      tunnel: [w381 w407] -> w110
      tunnel: [w381 w401] -> w107
      tunnel: [w381 w400] -> w109
      tunnel: [w381 w402] -> w108
      tunnel: [w381 w403] -> w97
      tunnel: [_ w398] -> w85
      tunnel: [_ w395] -> w83
      frame False {
        w381 = FALSE ("Initial E-Fuse")
        # "Select COM S0"
        n19 = local read "S_ValueC1(pF)"() -> (w387:dbl)
        n20 = local read "S_ValueC2(pF)"() -> (w386:dbl)
        n21 = local read "S_ValueC3(pF)"() -> (w385:dbl)
        n22 = call "WS1050_AD7747_Control_Cap_bank_Measure Ver1.0.vi"("Select Com Port"=w390, "S_Value C1"=w387, "S_Value C2"=w386, "S_Value C3"=w385, "errorin"=w392, "Push Button to Measue Cap"=TRUE) -> ("Com Port Out"=w389:refnum<visa-resource-name>, "C1_Mesa(pF)"=→"C1":dbl, "C2_Mesa(pF)"=→"C2":dbl, "C3_Mesa(pF)"=→"C3":dbl, "error out"=w391:errorcluster)  [unwired: 14 in, 3 out]
      }
      frame True {
        w425 = u16 0 items=["All Off", "Bank 1", "Bank 2", "Bank 3"] ("Ring")
        # "Initialize and Calibration"
        n23 = Format Into String(format string="%.;VOLT %f", "VDD \nSet Up") -> (resulting string=w415:string)  [unwired: 2 in, 1 out]
        n24 = VISA Write(VISA resource name=w414, write buffer=w415, error in (no error)=w413) -> (VISA resource name out=w411:refnum<visa-resource-name>, error out=w412:errorcluster)  [unwired: 1 out]
        n25 = Unbundle By Name("CMOS Setup") -> ("ECAL"=w407:bool, "Full Steps"=w401:bool, "Multi VPI"=w400:bool, "DVA"=w402:bool, "EFuse RB"=w406:bool, "Init RB"=w405:bool, "HS Test"=w403:bool)
        n26 = VISA Write(VISA resource name=w411, write buffer="OUTP 1;", error in (no error)=w412) -> (VISA resource name out=w408:refnum<visa-resource-name>, error out=w409:errorcluster)  [unwired: 1 out]
        n27 = call "WS105x_NI_6501_Relay_Control.vi"("Ring"=w425, "Relay_ 11"=TRUE, "error in (no error)"=w409, "Relay_ 10"=FALSE) -> ("error out"=w422:errorcluster)  [unwired: 2 in, 9 out]
        n28 = call "Delay.vi"("error in (no error)"=w422, "milliseconds to wait"=u32 100) -> ("error out"=w420:errorcluster)  [unwired: 9 in]
        n29 = Index Array(array=string[] ["07476F", "074776", "074777", "07479", "07477B", "07477C", "07477C"], index="Select CPV") -> (element=w398:string)
        n30 = call "WS1050_AD7747_Control_Cap_bank_Measure Ver1.0.vi"("Select Com Port"=w432, "errorin"=w420, "Push Button to Measue Cap"=TRUE, "Mode"=FALSE) -> ("Com Port Out"=w429:refnum<visa-resource-name>, "C1_Mesa(pF)"=w427:dbl, "C2_Mesa(pF)"=w426:dbl, "error out"=w431:errorcluster)  [unwired: 16 in, 4 out]
        n31 = Bundle("ECAL"=w407, "DVA"=w402, "Full Steps"=w401, "Multi VPI"=w400, "EFuse RB"=w406, "Init RB"=w405, "HS Test"=w403) -> (→"CMOS Out":T3)  [unwired: 1 in]
        n32 = case shown="1" "Select CPV" {
          tunnel: [35.0 40.25 41.0 42.5 44.0 50.0 55.0] -> w396
          frame 0, Default {
          }
          frame 1 {
          }
          frame 2 {
          }
          frame 3 {
          }
          frame 4 {
          }
          frame 5 {
          }
          frame 6 {
          }
        }
        n33 = Subtract(x=w427, y=w426) -> (x-y=w430:dbl)
        n34 = Absolute Value(x=w430) -> (abs(x)=w433:dbl)
        "Difference" <- w433
        n35 = Greater Or Equal?(x=w433, y="Allowed (pF)") -> (x >= y?=w436:bool)
        "Pass/Fail" <- w436
        n36 = case shown="True" w436 {
          tunnel: [w445 w448] -> w435
          tunnel: w436 -> [w445 w448]
          tunnel: w431 -> [w446 w447]
          tunnel: [w446 w447] -> w428
          frame False {
          }
          frame True {
            n37 = One Button Dialog(message="Please reinstall part") -> ()  [unwired: 1 in, 1 out]
          }
        }
        n38 = Number To Engineering String(4:w396) -> (0:w395:string)  [unwired: 3 in]
      }
    }
    n39 = Unbundle By Name(w195) -> ("Idd Low Limit (A)"=w190:dbl, "Idd High Limit (A)"=w111:dbl, "Idd Standby"=w101:dbl, "VSA Path1"=w182:string, "VSA"=w169:bool, "SWCyc"=w194:bool, "Test Name"=w166:string, "Loop Count"=w188:i32)  [unwired: 6 out]
    n40 = case shown="True" "Send" {
      tunnel: w87 -> [w462 w469]
      tunnel: w89 -> [w463 w464]
      tunnel: [w463 w468] -> w88
      tunnel: [w462 w467] -> w86
      frame False {
      }
      frame True {
        n41 = Index Array(array=string[] ["074000", "074040", "074820", "074800", "074044", "074040", "074776", "07476F", "074773", "07477B", "07477C", "074760", "074762", "074768", "07413B", "074100", "07423B", "074200", "07433B", "074300"], index="Manual CP Setting") -> (element=w465:string)
        n42 = VISA Write(VISA resource name=w469, write buffer=w465, error in (no error)=w464) -> (VISA resource name out=w467:refnum<visa-resource-name>, error out=w468:errorcluster)  [unwired: 1 out]
      }
    }
    n43 = String To Path(string=w182) -> (path=w174:path)
    n44 = Concatenate Strings("Test Name: " ("string"), "-----" ("string"), "Title", "\r\n", w166) -> (w179:string)
    n45 = case shown="0" w99 {
      tunnel: w179 -> [w206 _]
      tunnel: "TMN DC\\CAP Data Log File Path" -> [w205 _]
      tunnel: w88 -> [w204 w207]
      tunnel: [w203 w207] -> w98
      frame 0 {
        n46 = call "Save Config File.vi"("error in"=w204, "text"=w206, "base path"=w205) -> ("error out"=w203:errorcluster)  [unwired: 8 in]
      }
      frame 1, Default {
      }
    }
    n47 = Not(x=w197) -> (.not. x?=w189:bool)
    "POWER ON" <- w189
    n48 = case shown="True" w189 {
      tunnel: w141 -> [w368 w371]
      tunnel: [w368 w376] -> w144
      tunnel: w86 -> [w367 w372]
      tunnel: [w367 w373] -> w96
      frame False {
      }
      frame True {
        w369 = string[] [] ("EUSE Burn")
        w380 = "" ("EFuse 2")
        w378 = "0" ("Idd_Standby")
        n49 = local write "% Delta Cap"(0.0 ("% Delta Cap")) -> ()
        n50 = local write "I_stdby End"(w378) -> ()
        n51 = local write "IDD_Stdby"(w378) -> ()
        n52 = local write "IDD_All OFF"(w378) -> ()
        n53 = local write "IDD_All ON"(w378) -> ()
        n54 = local write "EFuse 1"(w380) -> ()
        n55 = local write "EFuse 2"(w380) -> ()
        n56 = call "Initialize RFFE.vi"("error in (no error)"=w371, "write buffer"="5", "Select Com Port"=w372) -> ("error out"=w375:errorcluster, "VISA resource name out"=w373:refnum<visa-resource-name>)  [unwired: 7 in]
        n57 = local write "RB All Regs Dump"(w369) -> ()
        n58 = local write "EUSE Burn"(w369) -> ()
        n59 = local write "Init EFuse RB"(w369) -> ()
        n60 = local write "CMin Delay_AST"(w369) -> ()
        n61 = local write "All Out"(string[] []) -> ()
        n62 = call "Delay.vi"("error in (no error)"=w375, "milliseconds to wait"=u32 100) -> ("error out"=w376:errorcluster)  [unwired: 9 in]
      }
    }
    n63 = case shown="True" "Calib\nSocket" {
      tunnel: w144 -> [w336 w360]
      tunnel: [w336 w340] -> w164
      tunnel: w118 -> [w334 w362]
      tunnel: w161 -> [w335 w346]
      tunnel: [w335 w341] -> w160
      tunnel: [w334 w358] -> w159
      frame False {
      }
      frame True {
        # "U9 = C3\nU7 = C1\nU8 = C2"
        n64 = flat-sequence {
          tunnel: [w364] -> w347
          tunnel: w360 -> [w364]
          tunnel: "Verify socket should be empty" ("message") -> [w363]
          frame #0 {
            n65 = One Button Dialog(message=w363) -> ()  [unwired: 1 in, 1 out]
          }
        }
        n66 = VISA Write(VISA resource name=w346, write buffer="VOLT 3.3;:OUTP 1", error in (no error)=w347) -> (VISA resource name out=w342:refnum<visa-resource-name>, error out=w344:errorcluster)  [unwired: 1 out]
        n67 = call "Delay.vi"("error in (no error)"=w344, "milliseconds to wait"=u32 250) -> ("error out"=w349:errorcluster)  [unwired: 9 in]
        n68 = call "WS1050_AD7747_Control_Cap_bank_Measure Ver1.0.vi"("Select Com Port"=w362, "errorin"=w349, "Push Button to Calibrate"=TRUE ("Push Button to Initialize AD7747")) -> ("Com Port Out"=w355:refnum<visa-resource-name>, "error out"=w356:errorcluster)  [unwired: 17 in, 6 out]
        n69 = call "WS1050_AD7747_Control_Cap_bank_Measure Ver1.0.vi"("Select Com Port"=w355, "errorin"=w356, "Push Button to Measue Cap"=TRUE) -> ("Com Port Out"=w358:refnum<visa-resource-name>, "C2(pF)"=→"S_ValueC2(pF)":dbl, "C1_Mesa(pF)"=→"C1Cal (pF)":dbl, "C2_Mesa(pF)"=→"C2Cal (pF)":dbl, "C3_Mesa(pF)"=→"C3Cal (pF)":dbl, "C1(pF)"=→"S_ValueC1(pF)":dbl, "C3(pF)"=→"S_ValueC3(pF)":dbl, "error out"=w337:errorcluster)  [unwired: 17 in]
        n70 = flat-sequence {
          tunnel: [w365] -> w339
          tunnel: w337 -> [w365]
          frame #0 {
            n71 = One Button Dialog(message="Socket Calibration Completed, Please insert DUT into the Socket") -> ()  [unwired: 1 in, 1 out]
          }
        }
        n72 = VISA Write(VISA resource name=w342, write buffer="VOLT 0.0", error in (no error)=w339) -> (VISA resource name out=w341:refnum<visa-resource-name>, error out=w340:errorcluster)  [unwired: 1 out]
      }
    }
    n73 = case shown="True" "Init AD7747" {
      tunnel: w159 -> [w290 w318]
      tunnel: [w291 w306] -> w121
      tunnel: w164 -> [w291 w311]
      tunnel: [w290 w300] -> w120
      tunnel: w160 -> [w289 w312]
      tunnel: [w289 w307] -> w104
      frame False {
      }
      frame True {
        w299 = string[] ["8", "9", "a"]
        # "Select COM S0"
        # "U9 = a = C3\nU7 = 8 = C1\nU8 = 9 = C2"
        n74 = VISA Write(VISA resource name=w312, write buffer="VOLT 3.3;:OUTP 1", error in (no error)=w311) -> (VISA resource name out=w308:refnum<visa-resource-name>, error out=w310:errorcluster)  [unwired: 1 out]
        n75 = call "Delay.vi"("error in (no error)"=w310, "milliseconds to wait"=u32 100) -> ("error out"=w314:errorcluster)  [unwired: 9 in]
        n76 = call "Initialize_PIC.vi"("error in (no error)"=w314, "baud rate"=u32 9600, "Select Com Port"=w318) -> ("error out"=w316:errorcluster, "VISA resource name out"=w317:refnum<visa-resource-name>)  [unwired: 7 in]
        n77 = for {
          tunnel: w317 -> [w331]
          tunnel: w299 -> [w327] mode=indexing
          tunnel: [w326] -> w302
          shift-right: [w328] -> w303
          shift-left: w316 -> [w330]
          n78 = call "AD7747_Setup.vi"("error in"=w330, "AD7747_Number"=w327, "Control"=w331) -> ("error out"=w329:errorcluster, "Control out"=w326:refnum<visa-resource-name>)  [unwired: 6 in, 1 out]
          n79 = call "Delay.vi"("error in (no error)"=w329, "milliseconds to wait"=u32 10) -> ("error out"=w328:errorcluster)  [unwired: 9 in]
        }
        n80 = for {
          tunnel: w303 -> [w324]
          tunnel: w302 -> [w323]
          tunnel: [w322] -> w301
          tunnel: [w321] -> w300
          tunnel: w299 -> [w320] mode=indexing
          tunnel: [w319] -> w298 mode=indexing
          n81 = call "WS1050_AD7747_MeasCAP_Ver1.1.vi"("error in (no error)"=w324, "AD7747_Number"=w320, "Control"=w323) -> ("error"=w322:errorcluster, "CAP (pF)"=w319:dbl, "Control out"=w321:refnum<visa-resource-name>)  [unwired: 4 in, 2 out]
        }
        n82 = Index Array(array=w298, index #1=0 ("index"), index #2=1 ("index"), index #3=2 ("index")) -> (element #1=→"C1(pF)":dbl, element #2=→"C2(pF)":dbl, element #3=→"C3(pF)":dbl)
        n83 = flat-sequence {
          tunnel: w301 -> [w332]
          tunnel: [w332] -> w305
          frame #0 {
            n84 = One Button Dialog(message="Initialize AD7747 completed!") -> ()  [unwired: 1 in, 1 out]
          }
        }
        n85 = VISA Write(VISA resource name=w308, write buffer="VOLT 0.0", error in (no error)=w305) -> (VISA resource name out=w307:refnum<visa-resource-name>, error out=w306:errorcluster)  [unwired: 1 out]
      }
    }
    n86 = Merge Errors(w121, w98) -> (w122:errorcluster)
    n87 = Wait Until Next ms Multiple(millisecond multiple=u32 50) -> ()  [unwired: 1 out]
    n88 = case shown="True" w145 {
      tunnel: [string[] ["n/a", "n/a", "n/a", "n/a", "n/a", "n/a", "n/a", "n/a", "n/a", "n/a"] w260] -> w143
      tunnel: w122 -> [w255 w257]
      tunnel: [w255 w264] -> w140
      tunnel: w96 -> [w253 w256]
      tunnel: [w253 w262] -> w124
      frame False {
      }
      frame True {
        n89 = for {
          tunnel: w257 -> [w267]
          tunnel: w256 -> [w266]
          tunnel: [w271] -> w262
          tunnel: [w272] -> w260 mode=indexing
          tunnel: string[] ["076000", "076100", "076200", "076300", "076400", "076500", "076600", "076700", "076800", "076900"] -> [w265] mode=indexing
          tunnel: [w273] -> w258
          w268 = u32 50 ("delay before read (ms)")
          n90 = call "RFFE Write Read Updated.vi"("VISA resource name"=w266, "write buffer"=w265, "delay before read (ms)"=w268, "error in (no error)"=w267) -> ("VISA resource name out"=w270:refnum<visa-resource-name>, "error out"=w269:errorcluster)  [unwired: 3 in, 2 out]
          n91 = call "RFFE Write Read Updated.vi"("VISA resource name"=w270, "write buffer"=w265, "delay before read (ms)"=w268, "error in (no error)"=w269) -> ("VISA resource name out"=w271:refnum<visa-resource-name>, "EFuse Read Back"=w272:string, "error out"=w273:errorcluster)  [unwired: 3 in, 1 out]
        }
        "Init EFuse RB" <- w260
        n92 = local write "Status"("Init EFUSE Read Back R1..." ("Status")) -> ()
        n93 = call "Delay.vi"("error in (no error)"=w258, "milliseconds to wait"=u32 10) -> ("error out"=w264:errorcluster)  [unwired: 9 in]
      }
    }
    n94 = local read "Title"() -> (w168:string)
    n95 = Bundle("Bench #"="Bench #", "Title"=w168, "Test Name"=w166, "Comment"="Comment") -> (w165:T5)  [unwired: 1 in]
    n96 = local read "Header Table"() -> (w131:string[][])
    n97 = Index Array(array=w131, index (row)=w132, index (col)=2 ("disabled index (col)")) -> (element=w129:string)
    n98 = Index Array(array=w131, index (row)=w132, index (col)=0 ("disabled index (col)")) -> (element=w135:string)
    n99 = Index Array(array=w131, index (row)=w132, index (col)=1 ("disabled index (col)")) -> (element=w133:string)
    n100 = case shown="True" w97 {
      tunnel: w140 -> [w240 w252]
      tunnel: [w240 w251] -> w139
      tunnel: "TMN DC\\CAP Data Log File Path" -> [_ w250]
      tunnel: ["OFF" w248] -> w128
      tunnel: w135 -> [_ w247]
      tunnel: w133 -> [_ w246]
      tunnel: w129 -> [_ w244]
      tunnel: w124 -> [w238 w243]
      tunnel: [w238 w242] -> w123
      tunnel: [TRUE ("P/F") w241] -> w112
      frame False {
      }
      frame True {
        n101 = local write "Status"("Handshaking R1....." ("Status")) -> ()
        n102 = call "WS1050 RFFE HS Check.vi"("file path (use dialog)"=w250, "Lot #"=w247, "Wafer #"=w246, "Reg1_Bit Cntrl"="Reg1_Bit Cntrl 2", "SN #"=w244, "RFFE COM Port"=w243, "error"=w252) -> ("VISA resource name out"=w242:refnum<visa-resource-name>, "s? t:f"=w248:string, "P/F"=w241:bool, "error out"=w251:errorcluster)  [unwired: 4 in, 1 out]
        "HS \nCheck" <- w241
      }
    }
    n103 = case shown="True" w125 {
      tunnel: [string[] ["n/a", "n/a"] w225] -> w127
      tunnel: w139 -> [w210 w229]
      tunnel: [w210 w212] -> w138
      tunnel: w123 -> [w208 w227]
      tunnel: [w208 w211] -> w137
      frame False {
      }
      frame True {
        w213 = u32 50 ("delay before read (ms)")
        w216 = "076500" ("write buffer")
        n104 = for {
          tunnel: w229 -> [w236]
          tunnel: string[] ["074920", "074900"] -> [w235] mode=indexing
          tunnel: w227 -> [w234]
          tunnel: [w231] -> w223
          tunnel: [w233] -> w224
          n105 = VISA Write(VISA resource name=w234, write buffer=w235, error in (no error)=w236) -> (VISA resource name out=w233:refnum<visa-resource-name>, error out=w232:errorcluster)  [unwired: 1 out]
          n106 = call "Delay.vi"("error in (no error)"=w232, "milliseconds to wait"=u32 50) -> ("error out"=w231:errorcluster)  [unwired: 9 in]
        }
        n107 = call "E-Fuse Readback.vi"("write buffer"=w216, "error in (no error)"=w223, "delay before read (ms)"=w213, "VISA resource name"=w224) -> ("error out"=w222:errorcluster, "VISA resource name out"=w221:refnum<visa-resource-name>)  [unwired: 5 in, 1 out]
        n108 = call "E-Fuse Readback.vi"("write buffer"=w216, "error in (no error)"=w222, "delay before read (ms)"=w213, "VISA resource name"=w221) -> ("error out"=w220:errorcluster, "VISA resource name out"=w219:refnum<visa-resource-name>)  [unwired: 5 in, 1 out]
        n109 = local write "Status"("EFUSE Read Back R5....." ("Status")) -> ()
        n110 = call "E-Fuse Readback.vi"("write buffer"=w216, "error in (no error)"=w220, "delay before read (ms)"=w213, "VISA resource name"=w219) -> ("error out"=w218:errorcluster, "EFuse Read Back"=w214:string, "VISA resource name out"=w217:refnum<visa-resource-name>)  [unwired: 5 in]
        "EFuse 1" <- w214
        n111 = call "E-Fuse Readback.vi"("write buffer"=w216, "error in (no error)"=w218, "delay before read (ms)"=w213, "VISA resource name"=w217) -> ("error out"=w212:errorcluster, "EFuse Read Back"=w215:string, "VISA resource name out"=w211:refnum<visa-resource-name>)  [unwired: 5 in]
        "EFuse 2" <- w215
        n112 = Build Array(w214, w215) -> (w225:string[])
      }
    }
    "After RB" <- w138
    n113 = case shown="True" w189 {
      tunnel: [w510 w533] -> w198
      tunnel: [FALSE ("Measure after Action?") w535] -> w196
      tunnel: [_ w536] -> w191
      tunnel: w138 -> [w508 w526]
      tunnel: [w508 w520] -> w156
      tunnel: w137 -> [w507 w524]
      tunnel: w150 -> [w506 w531]
      tunnel: [w507 w527] -> w149
      tunnel: [w506 w530] -> w148
      tunnel: w110 -> [_ w521]
      tunnel: w108 -> [_ w515]
      tunnel: ["n/a" w514] -> w106
      tunnel: ["n/a" w513] -> w105
      tunnel: w101 -> [_ w512]
      tunnel: w85 -> [_ w511]
      frame False {
        n114 = local read "IDD_Stdby"() -> (w510:string)
      }
      frame True {
        # "ECAL"
        # "Set DVD, CP Voltage"
        n115 = local write "Status"("Power on....." ("Status")) -> ()
        n116 = VISA Write(VISA resource name=w524, write buffer="074000", error in (no error)=w526) -> (VISA resource name out=w517:refnum<visa-resource-name>, error out=w525:errorcluster)  [unwired: 1 out]
        n117 = call "Delay.vi"("error in (no error)"=w525, "milliseconds to wait"=u32 100) -> ("error out"=w528:errorcluster)  [unwired: 9 in]
        n118 = call "Ke2000 Measurement.vi"("error in (no error)"=w528, "VISA resource name"=w531) -> ("error out"=w516:errorcluster, "Meas in micro"=w529:string, "VISA resource name out"=w530:refnum<visa-resource-name>)  [unwired: 4 in, 3 out]
        "IDD_Stdby" <- w529
        n119 = case shown="False" w515 {
          tunnel: [w543 w557] -> w519
          tunnel: [w544 w556] -> w518
          tunnel: w517 -> [w542 w555]
          tunnel: w516 -> [w541 w554]
          tunnel: ["OFF" "ON"] -> w514
          tunnel: w511 -> [w537 _]
          frame False {
            n120 = Insert Into Array(array=string[] ["074040", "074820"], new element=w537) -> (w538:string[])  [unwired: 1 in]
            n121 = for {
              tunnel: w542 -> [w551]
              tunnel: [w550] -> w544
              tunnel: w541 -> [w549]
              tunnel: [w547] -> w543
              tunnel: w538 -> [w546] mode=indexing
              n122 = VISA Write(VISA resource name=w551, write buffer=w546, error in (no error)=w549) -> (VISA resource name out=w550:refnum<visa-resource-name>, error out=w548:errorcluster)  [unwired: 1 out]
              n123 = call "Delay.vi"("error in (no error)"=w548, "milliseconds to wait"=u32 10) -> ("error out"=w547:errorcluster)  [unwired: 9 in]
            }
          }
          frame True {
            n124 = for {
              tunnel: w555 -> [w563]
              tunnel: [w562] -> w556
              tunnel: w554 -> [w561]
              tunnel: [w559] -> w557
              tunnel: string[] ["074040", "074800"] -> [w558] mode=indexing
              n125 = VISA Write(VISA resource name=w563, write buffer=w558, error in (no error)=w561) -> (VISA resource name out=w562:refnum<visa-resource-name>, error out=w560:errorcluster)  [unwired: 1 out]
              n126 = call "Delay.vi"("error in (no error)"=w560) -> ("error out"=w559:errorcluster)  [unwired: 10 in]
            }
          }
        }
        n127 = Fract/Exp String To Number(string=w529) -> (number=w532:dbl)  [unwired: 4 out]
        n128 = Greater Or Equal?(x=w532, y=w512) -> (x >= y?=w536:bool)
        n129 = case shown="False" w521 {
          tunnel: [w569 w579] -> w520
          tunnel: [w568 w584] -> w527
          tunnel: w519 -> [w567 w582]
          tunnel: w518 -> [w565 w581]
          tunnel: ["OFF" "ON"] -> w513
          frame False {
            n130 = for {
              tunnel: [w571] -> w569
              tunnel: w565 -> [w576]
              tunnel: [w575] -> w568
              tunnel: w567 -> [w574]
              tunnel: string[] ["074040", "074044"] -> [w573] mode=indexing
              n131 = VISA Write(VISA resource name=w576, write buffer=w573, error in (no error)=w574) -> (VISA resource name out=w575:refnum<visa-resource-name>, error out=w572:errorcluster)  [unwired: 1 out]
              n132 = call "Delay.vi"("error in (no error)"=w572, "milliseconds to wait"=u32 10) -> ("error out"=w571:errorcluster)  [unwired: 9 in]
            }
          }
          frame True {
            n133 = VISA Write(VISA resource name=w581, write buffer="074040", error in (no error)=w582) -> (VISA resource name out=w584:refnum<visa-resource-name>, error out=w578:errorcluster)  [unwired: 1 out]
            n134 = call "Delay.vi"("error in (no error)"=w578, "milliseconds to wait"=u32 10) -> ("error out"=w579:errorcluster)  [unwired: 9 in]
          }
        }
        n135 = case shown="True" w536 {
          selector: w536 -> [w587 _]
          tunnel: [w585 w590] -> w535
          tunnel: w529 -> [w586 w589]
          tunnel: [w586 w588] -> w533
          frame True {
            n136 = Not(x=w587) -> (.not. x?=w585:bool)
            n137 = local write "Pass /Fail?"(w585) -> ()
          }
          frame False {
            n138 = flat-sequence {
              tunnel: w589 -> [w592]
              tunnel: [w592] -> w588
              tunnel: [TRUE ("Pass/Fail")] -> w590
              frame #0 {
              }
            }
          }
        }
      }
    }
    "CHARGE \nPUMP ON" <- w196
    n139 = case shown="True" w196 {
      tunnel: [FALSE w489] -> w175
      tunnel: [_ w486] -> w192
      tunnel: w190 -> [_ w475]
      tunnel: w156 -> [w473 w478]
      tunnel: [w473 w481] -> w102
      tunnel: w149 -> [w471 w477]
      tunnel: w148 -> [w472 w483]
      tunnel: [w472 w482] -> w147
      tunnel: [w471 w477] -> w146
      tunnel: w111 -> [_ w476]
      frame False {
      }
      frame True {
        n140 = call "Delay.vi"("error in (no error)"=w478, "milliseconds to wait"=u32 100) -> ("error out"=w485:errorcluster)  [unwired: 9 in]
        n141 = local write "Status"("Charge Pump on....." ("Status")) -> ()
        n142 = call "Ke2000 Measurement.vi"("error in (no error)"=w485, "VISA resource name"=w483) -> ("error out"=w481:errorcluster, "Meas in micro"=w479:string, "VISA resource name out"=w482:refnum<visa-resource-name>)  [unwired: 4 in, 3 out]
        n143 = Fract/Exp String To Number(string=w479) -> (number=w480:dbl)  [unwired: 3 in, 1 out]
        n144 = In Range and Coerce(upper limit=w476, x=w480, lower limit=w475) -> (In Range?=w487:bool)  [unwired: 1 out]
        n145 = Not(x=w487) -> (.not. x?=w486:bool)
        n146 = case shown="True" w486 {
          selector: w486 -> [w491 _]
          tunnel: [w490 w492] -> w489
          frame True {
            n147 = Not(x=w491) -> (.not. x?=w490:bool)
            n148 = local write "Pass /Fail?"(w490) -> ()
          }
          frame False {
            n149 = flat-sequence {
              tunnel: [TRUE] -> w492
              frame #0 {
              }
            }
          }
        }
      }
    }
    n150 = And(x=w175, y=w194) -> (x .and. y?=w114:bool)
    "2K Cycles" <- w114
    n151 = Compound Arithmetic op=AND(w112, w114) -> (w113:bool)
    n152 = case shown="True" w113 {
      tunnel: [w452 w461] -> w117
      tunnel: w175 -> [w452 w461]
      tunnel: w188 -> [_ w456]
      tunnel: [w451 w459] -> w92
      tunnel: w102 -> [w451 w460]
      tunnel: w146 -> [w450 w453]
      tunnel: [w450 w458] -> w91
      frame False {
      }
      frame True {
        # "Loop Count 1 will have 2000 Cycles"
        n153 = Multiply(x=w456, y=2000 ("Number of Cycles")) -> (x*y=w454:i32)
        n154 = call "WS1050_PIC_RFFE_2K_Cycles.vi"("error in (no error)"=w460, "Initialize"=FALSE, "Number of Cycles"=w454, "VISA resource name 2"=w453) -> ("error out"=w459:errorcluster, "VISA resource name out"=w458:refnum<visa-resource-name>)  [unwired: 5 in, 1 out]
      }
    }
    n155 = And(x=w175, y=w169) -> (x .and. y?=w172:bool)
    "EXE SEQ" <- w172
    n156 = Compound Arithmetic op=AND(w112, w117) -> (w116:bool)
    n157 = Or(x=w191, y=w192) -> (x .or. y?=w171:bool)
    n158 = case shown="True" w172 {
      selector: w172 -> [_ w288]
      tunnel: [w285 w288] -> w170
      tunnel: w171 -> [w284 _]
      frame False {
        n159 = Select(t=FALSE ("status"), s=w284, f=TRUE ("status")) -> (s? t:f=w285:bool)
      }
      frame True {
      }
    }
    n160 = case shown="True" "Scope Set Up" {
      tunnel: w156 -> [w275 w276]
      tunnel: [w275 w283] -> w153
      tunnel: w93 -> [w274 w280]
      tunnel: [w274 w279] -> w155
      tunnel: "Save/Recal" -> [_ w278]
      tunnel: "Location" -> [_ w277]
      frame False {
      }
      frame True {
        n161 = call "DPO4034 Save Recall Setup.vi"("error in (no error)"=w276, "Save/Recall"=w278, "Location"=w277, "VISA resource name"=w280) -> ("error out"=w281:errorcluster, "VISA resource name out"=w279:refnum<visa-resource-name>)  [unwired: 6 in]
        n162 = call "Delay.vi"("error in (no error)"=w281, "milliseconds to wait"=u32 1000) -> ("error out"=w283:errorcluster)  [unwired: 9 in]
      }
    }
    n163 = case shown="True" w116 {
      selector: w116 -> [w612 _]
      tunnel: "TMN DC\\CAP Data Log File Path" -> [w615 w878]
      tunnel: w171 -> [w614 _]
      tunnel: w198 -> [w613 w846]
      tunnel: [w594 _] -> w185
      tunnel: w181 -> [w611 w873]
      tunnel: [w599 w761] -> w193
      tunnel: w184 -> [_ w860]
      tunnel: w92 -> [w608 w870]
      tunnel: w174 -> [_ w843]
      tunnel: w173 -> [w600 w728]
      tunnel: w170 -> [w610 _]
      tunnel: w169 -> [_ w861]
      tunnel: w165 -> [w609 w828]
      tunnel: [w598 w709] -> w163
      tunnel: [w600 w708] -> w162
      tunnel: [w599 w687] -> w158
      tunnel: [w596 w688] -> w157
      tunnel: w155 -> [w607 w872]
      tunnel: w153 -> [w605 w809]
      tunnel: [w607 w717] -> w152
      tunnel: "Comment" -> [_ w871]
      tunnel: w91 -> [w596 w856]
      tunnel: w147 -> [w595 w854]
      tunnel: w143 -> [w604 w818]
      tunnel: "Header Table" -> [w603 w827]
      tunnel: w128 -> [w602 w817]
      tunnel: w127 -> [w601 w816]
      tunnel: [w595 w806] -> w126
      tunnel: [w599 w687] -> w82
      tunnel: w120 -> [w597 w805]
      tunnel: [w597 w799] -> w119
      tunnel: w104 -> [w598 w789]
      tunnel: w107 -> [_ w733]
      tunnel: w109 -> [w593 w731]
      tunnel: w108 -> [_ w727]
      tunnel: w106 -> [_ w694]
      tunnel: w105 -> [_ w695]
      tunnel: w85 -> [_ w683]
      tunnel: w83 -> [_ w680]
      frame False {
        n164 = case shown="False" w610 {
          tunnel: w615 -> [_ w631]
          tunnel: w614 -> [_ w630]
          tunnel: w613 -> [_ w621]
          tunnel: [FALSE ("Pass/Fail?") w629] -> w594
          tunnel: w612 -> [_ w628]
          tunnel: w611 -> [_ w627]
          tunnel: w609 -> [_ w626]
          tunnel: w608 -> [w616 w625]
          tunnel: [w616 w624] -> w606
          tunnel: w604 -> [_ w623]
          tunnel: w603 -> [_ w622]
          tunnel: w602 -> [_ w620]
          tunnel: w601 -> [_ w619]
          tunnel: w593 -> [_ w618]
          frame True {
          }
          frame False {
            n165 = case shown="True" w630 {
              tunnel: w631 -> [_ w667]
              tunnel: [TRUE ("Pass/Fail?") w663] -> w629
              tunnel: w628 -> [_ _]
              tunnel: w627 -> [_ w662]
              tunnel: w626 -> [_ w655]
              tunnel: w625 -> [w632 w657]
              tunnel: [w632 w656] -> w624
              tunnel: w623 -> [_ w641]
              tunnel: w622 -> [_ w654]
              tunnel: w621 -> [_ w638]
              tunnel: w620 -> [_ w640]
              tunnel: w619 -> [_ w639]
              tunnel: w618 -> [_ w634]
              frame False {
              }
              frame True {
                w648 = 1 ("index (row)")
                n166 = Get Date/Time In Seconds() -> (seconds since 1Jan1904=w661:timestamp)
                n167 = Format Date/Time String(seconds (now)=w661, UTC format=FALSE) -> (date/time string=w659:string)  [unwired: 1 in]
                n168 = call <vilib>:"Space Constant.vi"() -> ("String"=w658:string)
                n169 = Index Array(array=w654, index (row) #1=w648, index (col) #1=0 ("index (row)"), index (row) #2=w648, index (col) #2=1 ("index (row)"), index (row) #3=w648, index (col) #3=2 ("disabled index (col)")) -> (element #1=w651:string, element #2=w650:string, element #3=w649:string)
                n170 = Match Pattern(string=w659, regular expression=w658) -> (before substring=w653:string, after substring=w652:string)  [unwired: 1 in, 2 out]
                n171 = for {
                  N: 168 -> [_]
                  tunnel: ["0" ("new element/subarray")] -> w636 mode=indexing
                }
                n172 = Build Array (concatenate)(w653, w652, w651, w650, w649, w641, w640, w639, w638) -> (w646:string[])
                n173 = for {
                  N: 54 -> [_]
                  tunnel: ["0" ("new element/subarray")] -> w643 mode=indexing
                }
                n174 = Insert Into Array(array=w646, new element=w636) -> (w645:string[])  [unwired: 1 in]
                n175 = call "WS1050_Full Step_RegDump_StepVPI_Ver1.4.vi"("ST Data Out"=w643, "CMin Delay_AST"=string[] ["0", "0", "0", "0", "0", "0", "0", "0", "0", "0", "0", "0", "0", "0", "0", "0"], "error in (no error)"=w657, "VPI_Result"=w634, "Lot"=w651, "Wafer"=w650, "TMN DC\\CAP Data Log File Path"=w667, "All Out"=w645, "Bin File Path"=w662, "Test Program"=w655, "EUSE Burn"=string[] ["n\\a", "n\\a"]) -> ("Bins"=w664:string, "error out"=w656:errorcluster)  [unwired: 12 in, 3 out]
                n176 = flat-sequence {
                  tunnel: w664 -> [w671]
                  tunnel: [w671] -> _
                  tunnel: [TRUE ("Pass/Fail?")] -> w663
                  frame #0 {
                  }
                }
              }
            }
          }
        }
        n177 = Merge Errors(w605, w606) -> (w599:errorcluster)
      }
      frame True {
        w790 = FALSE ("Relay_ 10")
        w791 = u16 0 items=["All Off", "Bank 1", "Bank 2", "Bank 3"] ("Ring")
        w807 = 1 ("index (row)")
        # "Save Data"
        # "Set CP for VSA and ST as\nScreen Parts.  Set DVA ON/OFF"
        # "CAP Meas"
        # "CAP Meas"
        # "RFFE"
        # "Ke2000"
        # "RFFE"
        # "Ke2000"
        n178 = flat-sequence {
          tunnel: w870 -> [w997]
          tunnel: w878 -> [w1021]
          tunnel: [w1021] -> w858
          tunnel: [w985] -> w857
          tunnel: w856 -> [w998]
          tunnel: [w999] -> w855
          tunnel: w854 -> [w1018]
          tunnel: [w1020] -> w852
          tunnel: ["Delay Cap Meas"] -> w850
          tunnel: [w1017] -> w849
          tunnel: w846 -> [w979]
          tunnel: w827 -> [w1003]
          tunnel: w818 -> [w1002]
          tunnel: w817 -> [w1001]
          tunnel: w816 -> [w1000]
          tunnel: w805 -> [w996]
          tunnel: [w986] -> w804
          tunnel: [w991] -> w785
          tunnel: [w995] -> w784
          tunnel: [w994] -> w781
          tunnel: ["Driver Name Full"] -> w780
          tunnel: ["Cmd Full"] -> w779
          tunnel: [w980] -> w735
          tunnel: [w981] -> w734
          tunnel: w733 -> [w991]
          tunnel: [w989] -> w719
          tunnel: w680 -> [w978]
          tunnel: [w1132] -> w869
          tunnel: [w1131] -> w868
          tunnel: [w1130] -> w867
          tunnel: [w1127] -> w866
          tunnel: w858 -> [w1133]
          tunnel: w857 -> [w1114]
          tunnel: w855 -> [w1116]
          tunnel: [w1126] -> w853
          tunnel: w852 -> [w1126]
          tunnel: w850 -> [w1125]
          tunnel: w849 -> [w1124]
          tunnel: [w1124] -> w848
          tunnel: [w1123] -> w847
          tunnel: [w1119] -> w838
          tunnel: w804 -> [w1117]
          tunnel: [w1115] -> w803
          tunnel: w785 -> [w1112]
          tunnel: w784 -> [w1111]
          tunnel: [w1109] -> w783
          tunnel: [w1112] -> w782
          tunnel: w781 -> [w1110]
          tunnel: w780 -> [w1106]
          tunnel: w779 -> [w1107]
          tunnel: [w1108] -> w778
          tunnel: [w1106] -> w777
          tunnel: [w1107] -> w776
          tunnel: [w1098] -> w772
          tunnel: [w1097] -> w768
          tunnel: w735 -> [w1096]
          tunnel: w734 -> [w1095]
          tunnel: w719 -> [w1094]
          tunnel: [w1094] -> w696
          tunnel: w869 -> [w1207]
          tunnel: w868 -> [w1224]
          tunnel: w867 -> [w1223]
          tunnel: w866 -> [w1179]
          tunnel: [w1219] -> w865
          tunnel: [w1218] -> w864
          tunnel: [w1217] -> w863
          tunnel: [w1216] -> w862
          tunnel: w853 -> [w1215]
          tunnel: [w1215] -> w851
          tunnel: w848 -> [w1214]
          tunnel: w847 -> [w1193]
          tunnel: [w1187] -> w845
          tunnel: [w1213] -> w844
          tunnel: w838 -> [w1210]
          tunnel: [w1209] -> w837
          tunnel: w803 -> [w1208]
          tunnel: [w1206] -> w802
          tunnel: w783 -> [w1204]
          tunnel: w782 -> [w1200]
          tunnel: w778 -> [w1203]
          tunnel: w777 -> [w1202]
          tunnel: w776 -> [w1201]
          tunnel: [w1200] -> w775
          tunnel: [w1197] -> w774
          tunnel: [w1196] -> w773
          tunnel: w772 -> [w1194]
          tunnel: [w1184] -> w771
          tunnel: w768 -> [w1181]
          tunnel: [w1181] -> w767
          tunnel: w696 -> [w1180]
          tunnel: [w1180] -> w692
          tunnel: w865 -> [w1311]
          tunnel: w864 -> [w1291]
          tunnel: w863 -> [w1307]
          tunnel: w862 -> [w1306]
          tunnel: [w1305] -> w760
          tunnel: [w1294] -> w759
          tunnel: [w1304] -> w758
          tunnel: [w1303] -> w757
          tunnel: w851 -> [w1302]
          tunnel: [w1302] -> w756
          tunnel: [w1301] -> w755
          tunnel: w845 -> [w1300]
          tunnel: w844 -> [w1283]
          tunnel: [w1277] -> w754
          tunnel: w837 -> [w1297]
          tunnel: [w1296] -> w753
          tunnel: w802 -> [w1295]
          tunnel: [w1293] -> w752
          tunnel: w775 -> [w1284]
          tunnel: w774 -> [w1289]
          tunnel: w773 -> [w1288]
          tunnel: w771 -> [w1287]
          tunnel: [w1272] -> w751
          tunnel: [w1284] -> w750
          tunnel: w767 -> [w1275]
          tunnel: w692 -> [w1269]
          tunnel: [w1269] -> w691
          tunnel: w760 -> [w1373]
          tunnel: [w1373] -> w749
          tunnel: w759 -> [w1356]
          tunnel: w758 -> [w1377]
          tunnel: [w1377] -> w748
          tunnel: w757 -> [w1374]
          tunnel: w756 -> [w1361]
          tunnel: [w1361] -> w747
          tunnel: w755 -> [w1368]
          tunnel: w754 -> [w1372]
          tunnel: w753 -> [w1376]
          tunnel: [w1376] -> w746
          tunnel: w752 -> [w1359]
          tunnel: [w1359] -> w745
          tunnel: w751 -> [w1375]
          tunnel: [w1375] -> w744
          tunnel: w750 -> [w1357]
          tunnel: [w1357] -> w743
          tunnel: [w1360] -> w742
          tunnel: [w1355] -> w741
          tunnel: [w1367] -> w740
          tunnel: [w1366] -> w739
          tunnel: [w1365] -> w738
          tunnel: [w1364] -> w737
          tunnel: [w1363] -> w736
          tunnel: [w1358] -> w732
          tunnel: w731 -> [w1358]
          tunnel: w691 -> [w1353]
          tunnel: [w1353] -> w690
          tunnel: w683 -> [w1352]
          tunnel: [w1352] -> w682
          tunnel: [w1413] -> w792
          tunnel: [w1406] -> w703
          tunnel: [w1405] -> w721
          tunnel: [w1408] -> w793
          tunnel: [w1412] -> w770
          tunnel: [w1396] -> w769
          tunnel: [w1385] -> w729
          tunnel: [w1411] -> w724
          tunnel: [w1410] -> w723
          tunnel: [w1409] -> w722
          tunnel: [w1407] -> w730
          tunnel: w732 -> [w1397]
          tunnel: w749 -> [w1398]
          tunnel: w748 -> [w1385]
          tunnel: w747 -> [w1403]
          tunnel: w746 -> [w1413]
          tunnel: w745 -> [w1402]
          tunnel: w744 -> [w1412]
          tunnel: w743 -> [w1396]
          tunnel: w742 -> [w1404]
          tunnel: w741 -> [w1401]
          tunnel: w740 -> [w1411]
          tunnel: w739 -> [w1410]
          tunnel: w738 -> [w1409]
          tunnel: w737 -> [w1400]
          tunnel: w736 -> [w1399]
          tunnel: ["S-Time"] -> w726
          tunnel: [w1385] -> w725
          tunnel: ["CMin/Delay"] -> w716
          tunnel: [w1393] -> w707
          tunnel: [w1392] -> w706
          tunnel: [w1391] -> w693
          tunnel: w690 -> [w1390]
          tunnel: [w1390] -> w689
          tunnel: w682 -> [w1387]
          tunnel: [w1386] -> w681
          frame #0 {
            w1014 = 1 ("index (row)")
            # "IDD @ 40V"
            n179 = stacked-sequence {
              seq-local: [w1040 _ _] -> [_ w1062 _]
              seq-local: [w1031 _ _] -> [_ w1064 _]
              seq-local: [w1033 _ _] -> [_ w1065 _]
              seq-local: [_ w1055 _] -> [_ _ w1085]
              seq-local: [_ w1053 _] -> [_ _ w1080]
              seq-local: [_ w1057 _] -> [_ _ w1079]
              seq-local: [w1029 _ _] -> [_ w1051 _]
              seq-local: [_ w1051 _] -> [_ _ w1072]
              tunnel: w997 -> [w1043 _ _]
              tunnel: [_ _ w1082] -> w985
              tunnel: w1018 -> [w1042 _ _]
              tunnel: [w1041 _ _] -> w980
              tunnel: [_ w1063 _] -> w981
              tunnel: [_ _ w1079] -> w1020
              tunnel: w998 -> [w1039 _ _]
              tunnel: "Delay Cap Meas" -> [w1036 w1059 _]
              tunnel: [_ _ w1091] -> w982
              tunnel: [_ _ w1090] -> w983
              tunnel: [_ _ w1089] -> w984
              tunnel: [_ _ w1081] -> w999
              tunnel: [_ _ w1080] -> w986
              tunnel: w996 -> [w1029 _ _]
              tunnel: "RB All Regs" -> [w1030 w1052 _]
              tunnel: [_ w1050 _] -> w988
              tunnel: [w1028 _ _] -> w987
              frame #0 {
                n180 = for {
                  tunnel: w1043 -> [w1049]
                  tunnel: [w1048] -> w1032
                  tunnel: w1039 -> [w1047]
                  tunnel: [w1046] -> w1037
                  tunnel: string[] ["07413B", "07423B", "07433B"] -> [w1045] mode=indexing
                  n181 = VISA Write(VISA resource name=w1047, write buffer=w1045, error in (no error)=w1049) -> (VISA resource name out=w1048:refnum<visa-resource-name>, error out=w1046:errorcluster)  [unwired: 1 out]
                  n182 = Wait Until Next ms Multiple(millisecond multiple=u32 50) -> ()  [unwired: 1 out]
                }
                n183 = call "Delay.vi"("error in (no error)"=w1037, "milliseconds to wait"=w1036) -> ("error out"=w1038:errorcluster)  [unwired: 9 in]
                n184 = call "Ke2000 Measurement.vi"("error in (no error)"=w1038, "VISA resource name"=w1042) -> ("error out"=w1034:errorcluster, "Meas in micro"=w1041:string, "VISA resource name out"=w1040:refnum<visa-resource-name>)  [unwired: 4 in, 3 out]
                n185 = call "RFFE_Readback All Registers.vi"("error out"=w1034, "RB All Regs"=w1030, "VISA IN"=w1032) -> ("error out 2"=w1033:errorcluster, "ALL Regs RB"=w1028:string[], "VISA OUT"=w1031:refnum<visa-resource-name>)  [unwired: 6 in]
              }
              frame #1 {
                n186 = for {
                  tunnel: w1065 -> [w1071]
                  tunnel: w1064 -> [w1070]
                  tunnel: [w1069] -> w1054
                  tunnel: [w1068] -> w1060
                  tunnel: string[] ["074100", "074200", "074300"] -> [w1066] mode=indexing
                  n187 = VISA Write(VISA resource name=w1070, write buffer=w1066, error in (no error)=w1071) -> (VISA resource name out=w1069:refnum<visa-resource-name>, error out=w1068:errorcluster)  [unwired: 1 out]
                  n188 = Wait Until Next ms Multiple(millisecond multiple=u32 50) -> ()  [unwired: 1 out]
                }
                n189 = call "Delay.vi"("error in (no error)"=w1060, "milliseconds to wait"=w1059) -> ("error out"=w1061:errorcluster)  [unwired: 9 in]
                n190 = call "Ke2000 Measurement.vi"("error in (no error)"=w1061, "VISA resource name"=w1062) -> ("error out"=w1056:errorcluster, "Meas in micro"=w1063:string, "VISA resource name out"=w1057:refnum<visa-resource-name>)  [unwired: 4 in, 3 out]
                n191 = call "RFFE_Readback All Registers.vi"("error out"=w1056, "RB All Regs"=w1052, "VISA IN"=w1054) -> ("error out 2"=w1055:errorcluster, "ALL Regs RB"=w1050:string[], "VISA OUT"=w1053:refnum<visa-resource-name>)  [unwired: 6 in]
              }
              frame #2 {
                n192 = local read "S_ValueC2(pF)"() -> (w1074:dbl)
                n193 = local read "S_ValueC1(pF)"() -> (w1075:dbl)
                n194 = local read "S_ValueC3(pF)"() -> (w1073:dbl)
                n195 = call "WS1050_AD7747_MeasCAP_Ver1.1.vi"("error in (no error)"=w1085, "OFFSet Cal"=w1075, "AD7747_Number"="8", "Control"=w1072) -> ("error"=w1083:errorcluster, 1:"CAP (pF)"=w1091:string, 2:"CAP (pF)"=→"CMin C1(pF)":dbl, "Control out"=w1084:refnum<visa-resource-name>)  [unwired: 3 in, 1 out]
                n196 = call "WS1050_AD7747_MeasCAP_Ver1.1.vi"("error in (no error)"=w1083, "OFFSet Cal"=w1074, "AD7747_Number"="9", "Control"=w1084) -> ("error"=w1093:errorcluster, 1:"CAP (pF)"=w1090:string, 2:"CAP (pF)"=→"CMin C2(pF)":dbl, "Control out"=w1092:refnum<visa-resource-name>)  [unwired: 3 in, 1 out]
                n197 = call "WS1050_AD7747_MeasCAP_Ver1.1.vi"("error in (no error)"=w1093, "OFFSet Cal"=w1073, "AD7747_Number"="a", "Control"=w1092) -> ("error"=w1082:errorcluster, 1:"CAP (pF)"=w1089:string, 2:"CAP (pF)"=→"CMin C3(pF)":dbl, "Control out"=w1081:refnum<visa-resource-name>)  [unwired: 3 in, 1 out]
              }
            }
            n198 = Index Array(array=w1003, index (row)=w1014, index (col)=0 ("disabled index (col)")) -> (element=w1010:string)
            "Lot" <- w1010
            n199 = Index Array(array=w1003, index (row)=w1014, index (col)=1) -> (element=w1011:string)
            "Wafer" <- w1011
            n200 = Index Array(array=w1003, index (row)=w1014, index (col)=2) -> (element=w1012:string)
            n201 = Get Date/Time In Seconds() -> (seconds since 1Jan1904=w1006:timestamp)
            n202 = Format Date/Time String(seconds (now)=w1006, UTC format=FALSE) -> (date/time string=w1007:string)  [unwired: 1 out]
            n203 = call <vilib>:"Space Constant.vi"() -> ("String"=w1008:string)
            n204 = for {
              tunnel: "Driver Name Full" -> [w1025] mode=indexing
              tunnel: [w1026] -> w995 mode=indexing
              tunnel: "Cmd Full" -> [w1023] mode=indexing
              tunnel: [w1022] -> w994 mode=indexing
              n205 = Concatenate Strings("C1_" ("string"), w1025) -> (w1026:string)
              n206 = Concatenate Strings("0741" ("string"), w1023) -> (w1022:string)
            }
            n207 = Match Pattern(string=w1007, regular expression=w1008) -> (before substring=w1005:string, after substring=w1004:string)  [unwired: 3 out]
            n208 = Insert Into Array(array=w987, new element=w988) -> (w989:string[])  [unwired: 1 in]
            n209 = Build Array (concatenate)(w1005, w1004, w1010, w1011, w1012, w1002, w1001, w1000, w978, w979, w980, w981, w982, w983, w984) -> (w1017:string[])
          }
          frame #1 {
            # "CAP Mease"
            n210 = case shown="False" w1112 {
              tunnel: ["C1" w1150] -> w1100
              tunnel: ["C1 Cmd" w1149] -> w1118
              tunnel: w1114 -> [w1148 w1151]
              tunnel: [w1148 w1151] -> w1113
              tunnel: w1111 -> [_ w1150]
              tunnel: w1110 -> [_ w1149]
              frame False {
              }
              frame True {
              }
            }
            n211 = Split 1D Array(array=w1106, index=59) -> (first subarray=w1104:string[])  [unwired: 1 out]
            n212 = Delete From Array(array=w1104, index=58) -> (array with subset deleted=w1097:string[])  [unwired: 1 in, 1 out]
            n213 = property on="Sequence" class="LstBox (strict)"(error in=w1113, "Item Names"=w1100) -> (error out=w1129:errorcluster)  [unwired: 1 in, 1 out]
            n214 = for {
              tunnel: w1097 -> [w1139] mode=indexing
              tunnel: [w1138] -> w1102 mode=indexing
              tunnel: w1097 -> [w1136] mode=indexing
              tunnel: [w1134] -> w1101 mode=indexing
              n215 = Concatenate Strings("Delta_C1_" ("string"), w1139) -> (w1138:string)
              n216 = Concatenate Strings("RTZ_C1_" ("string"), w1136) -> (w1134:string)
            }
            n217 = property on="Sequence" class="LstBox (strict)"(error in=w1129) -> (error out=w1121:errorcluster, "Item Names"=w1128:string[])  [unwired: 1 in, 1 out]
            n218 = Array Size(array=w1128) -> (size(s)=w1122:i32)
            n219 = for {
              N: w1122 -> [_]
              tunnel: w1133 -> [w1173]
              tunnel: [w1173] -> w1131
              tunnel: [w1169] -> w1132
              tunnel: w1125 -> [w1167]
              tunnel: [w1167] -> w1130
              tunnel: w1118 -> [w1172] mode=indexing
              tunnel: w1117 -> [w1171]
              tunnel: w1121 -> [w1170]
              tunnel: [w1160] -> w1123 mode=indexing
              tunnel: [w1162] -> w1127
              shift-right: [w1159] -> _
              shift-left: dbl[] [0.0] -> [w1161]
              tunnel: [w1157] -> w1119
              tunnel: w1116 -> [w1156]
              tunnel: [w1155] -> w1115
              i -> [w1158]
              n220 = VISA Write(VISA resource name=w1171, write buffer=w1172, error in (no error)=w1170) -> (VISA resource name out=w1155:refnum<visa-resource-name>, error out=w1168:errorcluster)  [unwired: 1 out]
              n221 = local read "S_ValueC1(pF)"() -> (w1154:dbl)
              n222 = local read "CMin C1(pF)"() -> (w1153:dbl)
              n223 = call "Delay.vi"("error in (no error)"=w1168, "milliseconds to wait"=w1167) -> ("error out"=w1164:errorcluster)  [unwired: 9 in]
              n224 = call "WS1050_AD7747_MeasCAP_Ver1.1.vi"("error in (no error)"=w1164, "OFFSet Cal"=w1154, "AD7747_Number"="8", "Control"=w1156) -> ("error"=w1166:errorcluster, "CAP (pF)"=w1160:string, "Control out"=w1169:refnum<visa-resource-name>)  [unwired: 3 in, 2 out]
              n225 = Fract/Exp String To Number(string=w1160) -> (number=w1152:dbl)  [unwired: 3 in, 1 out]
              n226 = call "Delay.vi"("error in (no error)"=w1166, "milliseconds to wait"=u32 10) -> ("error out"=w1162:errorcluster)  [unwired: 9 in]
              n227 = case shown="58" w1158 {
                tunnel: w1152 -> [_ w1178]
                tunnel: [w1175 w1177] -> w1157
                tunnel: w1153 -> [_ w1176]
                frame 0, Default {
                  n228 = local read "Delta_C1(pF)"() -> (w1175:dbl)
                }
                frame 58 {
                  n229 = Subtract(x=w1178, y=w1176) -> (x-y=w1177:dbl)
                  "Delta_C1(pF)" <- w1177
                }
              }
              n230 = local write "Status"("Testing C1....." ("Status")) -> ()
              n231 = Build Array (concatenate)(w1161, w1152) -> (w1159:dbl[])
              "C1 Graph" <- w1159
              "Sequence" <- w1158
            }
            "Bank C1" <- w1123
            n232 = Insert Into Array(array=w1102, new element=w1101) -> (w1099:string[])  [unwired: 1 in]
            n233 = for {
              tunnel: w1106 -> [w1143] mode=indexing
              tunnel: [w1144] -> w1109 mode=indexing
              tunnel: w1107 -> [w1141] mode=indexing
              tunnel: [w1140] -> w1108 mode=indexing
              n234 = Concatenate Strings("C2_" ("string"), w1143) -> (w1144:string)
              n235 = Concatenate Strings("0742" ("string"), w1141) -> (w1140:string)
            }
            n236 = Insert Into Array(array=w1100, new element=w1099) -> (w1098:string[])  [unwired: 1 in]
            "IDD_All ON" <- w1096
            "IDD_All OFF" <- w1095
            "RB All Regs Dump" <- w1094
          }
          frame #2 {
            n237 = local read "CMin C1(pF)"() -> (w1192:dbl)
            n238 = Insert Into Array(array=w1214, new element=w1193) -> (w1189:string[])  [unwired: 1 in]
            n239 = case shown="False" w1200 {
              tunnel: ["C2L" w1241] -> w1195
              tunnel: w1179 -> [w1238 w1242]
              tunnel: [w1238 w1242] -> w1199
              tunnel: ["WS1050 C2L Cmd" w1240] -> w1205
              tunnel: w1204 -> [_ w1241]
              tunnel: w1203 -> [_ w1240]
              frame False {
              }
              frame True {
              }
            }
            n240 = call "WS1050 Delta C_RTZ Ver1.0.vi"("CMin_C1"=w1192, "Bank C1"=w1193) -> ("C1_RTZ"=w1191:string[], "Delta C(pF)"=w1190:string[])  [unwired: 7 in, 1 out]
            n241 = Insert Into Array(array=w1194, new element=w1195) -> (w1182:string[])  [unwired: 1 in]
            n242 = property on="Sequence" class="LstBox (strict)"(error in=w1199, "Item Names"=w1195) -> (error out=w1221:errorcluster)  [unwired: 1 in, 1 out]
            n243 = Insert Into Array(array=w1190, new element=w1191) -> (w1188:string[])  [unwired: 1 in]
            n244 = for {
              tunnel: w1181 -> [w1230] mode=indexing
              tunnel: [w1229] -> w1185 mode=indexing
              tunnel: w1181 -> [w1227] mode=indexing
              tunnel: [w1225] -> w1186 mode=indexing
              n245 = Concatenate Strings("Delta_C2_" ("string"), w1230) -> (w1229:string)
              n246 = Concatenate Strings("RTZ_C2_" ("string"), w1227) -> (w1225:string)
            }
            n247 = property on="Sequence" class="LstBox (strict)"(error in=w1221) -> (error out=w1198:errorcluster, "Item Names"=w1222:string[])  [unwired: 1 in, 1 out]
            n248 = Insert Into Array(array=w1189, new element=w1188) -> (w1187:string[])  [unwired: 1 in]
            n249 = Array Size(array=w1222) -> (size(s)=w1220:i32)
            n250 = for {
              N: w1220 -> [_]
              tunnel: w1224 -> [w1263]
              tunnel: [w1263] -> w1219
              tunnel: w1223 -> [w1258]
              tunnel: [w1258] -> w1217
              tunnel: w1205 -> [w1262] mode=indexing
              tunnel: w1208 -> [w1261]
              tunnel: [w1252] -> w1213 mode=indexing
              tunnel: [w1254] -> w1218
              tunnel: w1198 -> [w1257]
              tunnel: [w1245] -> w1216
              shift-right: [w1250] -> _
              shift-left: dbl[] [0.0] -> [w1251]
              tunnel: [w1247] -> w1211
              tunnel: w1207 -> [w1246]
              tunnel: [w1244] -> w1206
              i -> [w1249]
              n251 = VISA Write(VISA resource name=w1261, write buffer=w1262, error in (no error)=w1257) -> (VISA resource name out=w1245:refnum<visa-resource-name>, error out=w1259:errorcluster)  [unwired: 1 out]
              n252 = local read "S_ValueC2(pF)"() -> (w1243:dbl)
              n253 = call "Delay.vi"("error in (no error)"=w1259, "milliseconds to wait"=w1258) -> ("error out"=w1260:errorcluster)  [unwired: 9 in]
              n254 = local write "Sequence"(w1249) -> ()
              n255 = call "WS1050_AD7747_MeasCAP_Ver1.1.vi"("error in (no error)"=w1260, "OFFSet Cal"=w1243, "AD7747_Number"="9" ("CNTR2_AD7747"), "Control"=w1246) -> ("error"=w1256:errorcluster, "CAP (pF)"=w1252:string, "Control out"=w1244:refnum<visa-resource-name>)  [unwired: 3 in, 2 out]
              n256 = Fract/Exp String To Number(string=w1252) -> (number=w1248:dbl)  [unwired: 3 in, 1 out]
              n257 = case shown="58" w1249 {
                tunnel: w1248 -> [_ w1268]
                tunnel: [w1265 w1267] -> w1247
                frame 0, Default {
                  n258 = local read "Delta_C2(pF)"() -> (w1265:dbl)
                }
                frame 58 {
                  n259 = local read "CMin C2(pF)"() -> (w1266:dbl)
                  n260 = Subtract(x=w1268, y=w1266) -> (x-y=w1267:dbl)
                  "Delta_C2(pF)" <- w1267
                }
              }
              n261 = local write "Status"("Testing C2....." ("Status")) -> ()
              n262 = call "Delay.vi"("error in (no error)"=w1256, "milliseconds to wait"=u32 10) -> ("error out"=w1254:errorcluster)  [unwired: 9 in]
              n263 = Build Array (concatenate)(w1251, w1248) -> (w1250:dbl[])
              "C2 Graph" <- w1250
            }
            n264 = Insert Into Array(array=w1185, new element=w1186) -> (w1183:string[])  [unwired: 1 in]
            n265 = for {
              tunnel: w1202 -> [w1234] mode=indexing
              tunnel: [w1235] -> w1197 mode=indexing
              tunnel: w1201 -> [w1232] mode=indexing
              tunnel: [w1231] -> w1196 mode=indexing
              n266 = Concatenate Strings("C3_" ("string"), w1234) -> (w1235:string)
              n267 = Concatenate Strings("0743" ("string"), w1232) -> (w1231:string)
            }
            n268 = Insert Into Array(array=w1182, new element=w1183) -> (w1184:string[])  [unwired: 1 in]
            n269 = Add(x=w1211, y=w1210) -> (x+y=w1209:dbl)
          }
          frame #3 {
            # "RFFE"
            n270 = local read "CMin C2(pF)"() -> (w1282:dbl)
            n271 = Insert Into Array(array=w1300, new element=w1283) -> (w1279:string[])  [unwired: 1 in]
            n272 = case shown="True" w1284 {
              tunnel: ["C3L" w1324] -> w1285
              tunnel: ["WS1050 C3L Cmd" w1323] -> w1292
              tunnel: w1291 -> [w1319 w1325]
              tunnel: [w1319 w1325] -> w1290
              tunnel: w1289 -> [_ w1324]
              tunnel: w1288 -> [_ w1323]
              tunnel: w1287 -> [w1318 w1322]
              tunnel: [w1318 w1322] -> w1286
              frame False {
              }
              frame True {
              }
            }
            n273 = call "WS1050 Delta C_RTZ Ver1.0.vi"("CMin_C1"=w1282, "Bank C1"=w1283) -> ("C1_RTZ"=w1280:string[], "Delta C(pF)"=w1281:string[])  [unwired: 7 in, 1 out]
            n274 = Insert Into Array(array=w1281, new element=w1280) -> (w1278:string[])  [unwired: 1 in]
            n275 = Insert Into Array(array=w1286, new element=w1285) -> (w1270:string[])  [unwired: 1 in]
            n276 = property on="Sequence" class="LstBox (strict)"(error in=w1290, "Item Names"=w1285) -> (error out=w1310:errorcluster)  [unwired: 1 in, 1 out]
            n277 = Insert Into Array(array=w1279, new element=w1278) -> (w1277:string[])  [unwired: 1 in]
            n278 = for {
              tunnel: w1275 -> [w1317] mode=indexing
              tunnel: [w1316] -> w1273 mode=indexing
              tunnel: [w1313] -> w1274 mode=indexing
              tunnel: w1275 -> [w1312] mode=indexing
              n279 = Concatenate Strings("Delta_C3_" ("string"), w1317) -> (w1316:string)
              n280 = Concatenate Strings("RTZ_C3_" ("string"), w1312) -> (w1313:string)
            }
            n281 = property on="Sequence" class="LstBox (strict)"(error in=w1310) -> (error out=w1276:errorcluster, "Item Names"=w1309:string[])  [unwired: 1 in, 1 out]
            n282 = Insert Into Array(array=w1273, new element=w1274) -> (w1271:string[])  [unwired: 1 in]
            n283 = Array Size(array=w1309) -> (size(s)=w1308:i32)
            n284 = for {
              N: w1308 -> [_]
              tunnel: w1311 -> [w1346]
              tunnel: [w1346] -> w1304
              tunnel: w1307 -> [w1341]
              tunnel: [w1341] -> w1305
              tunnel: w1292 -> [w1345] mode=indexing
              tunnel: w1306 -> [w1344]
              tunnel: [w1334] -> w1301 mode=indexing
              tunnel: [w1336] -> w1303
              tunnel: [w1339] -> w1293
              tunnel: w1276 -> [w1340]
              shift-right: [w1332] -> _
              shift-left: dbl[] [0.0] -> [w1333]
              tunnel: [w1329] -> w1298
              tunnel: w1295 -> [w1328]
              tunnel: [w1327] -> w1294
              i -> [w1331]
              n285 = VISA Write(VISA resource name=w1344, write buffer=w1345, error in (no error)=w1340) -> (VISA resource name out=w1327:refnum<visa-resource-name>, error out=w1342:errorcluster)  [unwired: 1 out]
              n286 = local read "S_ValueC3(pF)"() -> (w1326:dbl)
              n287 = local write "Sequence"(w1331) -> ()
              n288 = call "Delay.vi"("error in (no error)"=w1342, "milliseconds to wait"=w1341) -> ("error out"=w1343:errorcluster)  [unwired: 9 in]
              n289 = call "WS1050_AD7747_MeasCAP_Ver1.1.vi"("error in (no error)"=w1343, "OFFSet Cal"=w1326, "AD7747_Number"="a" ("CNTR1_AD7747"), "Control"=w1328) -> ("error"=w1338:errorcluster, "CAP (pF)"=w1334:string, "Control out"=w1339:refnum<visa-resource-name>)  [unwired: 3 in, 2 out]
              n290 = local write "Status"("Testing C3....." ("Status")) -> ()
              n291 = Fract/Exp String To Number(string=w1334) -> (number=w1330:dbl)  [unwired: 3 in, 1 out]
              n292 = case shown="58" w1331 {
                tunnel: w1330 -> [_ w1351]
                tunnel: [w1348 w1350] -> w1329
                frame 0, Default {
                  n293 = local read "Delta_C3(pF)"() -> (w1348:dbl)
                }
                frame 58 {
                  n294 = local read "CMin C3(pF)"() -> (w1349:dbl)
                  n295 = Subtract(x=w1351, y=w1349) -> (x-y=w1350:dbl)
                  "Delta_C3(pF)" <- w1350
                }
              }
              n296 = call "Delay.vi"("error in (no error)"=w1338, "milliseconds to wait"=u32 10) -> ("error out"=w1336:errorcluster)  [unwired: 9 in]
              n297 = Build Array (concatenate)(w1333, w1330) -> (w1332:dbl[])
              "C3 Graph" <- w1332
            }
            n298 = Insert Into Array(array=w1270, new element=w1271) -> (w1272:string[])  [unwired: 1 in]
            n299 = Add(x=w1298, y=w1297) -> (x+y=w1296:dbl)
          }
          frame #4 {
            # "Disable ECAL/DVA"
            # "23.75V"
            n300 = local read "CMin C3(pF)"() -> (w1369:dbl)
            n301 = Insert Into Array(array=w1372, new element=w1368) -> (w1364:string[])  [unwired: 1 in]
            n302 = local write "VPIData Out"(string[][] [] ("VPIData Out")) -> ()
            n303 = for {
              tunnel: string[] ["074820", "074044"] -> [w1384] mode=indexing
              tunnel: w1374 -> [w1383]
              tunnel: [w1381] -> w1360
              tunnel: w1356 -> [w1379]
              tunnel: [w1378] -> w1355
              n304 = VISA Write(VISA resource name=w1379, write buffer=w1384, error in (no error)=w1383) -> (VISA resource name out=w1378:refnum<visa-resource-name>, error out=w1382:errorcluster)  [unwired: 1 out]
              n305 = call "Delay.vi"("error in (no error)"=w1382, "milliseconds to wait"=u32 10) -> ("error out"=w1381:errorcluster)  [unwired: 9 in]
            }
            n306 = local read "S_ValueC1(pF)"() -> (w1367:dbl)
            n307 = local read "S_ValueC2(pF)"() -> (w1366:dbl)
            n308 = local read "S_ValueC3(pF)"() -> (w1365:dbl)
            n309 = call "WS1050 Delta C_RTZ Ver1.0.vi"("CMin_C1"=w1369, "Bank C1"=w1368) -> ("C1_RTZ"=w1370:string[], "Delta C(pF)"=w1371:string[])  [unwired: 7 in, 1 out]
            n310 = Insert Into Array(array=w1371, new element=w1370) -> (w1363:string[])  [unwired: 1 in]
          }
          frame #5 {
            # "RFFE"
            # "Ke2000"
            n311 = case shown="True" w1397 {
              tunnel: w1404 -> [w1417 w1448]
              tunnel: w1403 -> [w1423 w1447]
              tunnel: w1402 -> [w1421 w1446]
              tunnel: w1401 -> [w1422 w1445]
              tunnel: [w1416 w1444] -> w1406
              tunnel: [w1423 w1443] -> w1408
              tunnel: [w1422 w1442] -> w1407
              tunnel: [w1421 w1441] -> w1405
              tunnel: w1398 -> [_ w1439]
              tunnel: w1409 -> [_ w1434]
              tunnel: w1410 -> [_ w1433]
              tunnel: w1411 -> [_ w1432]
              tunnel: [w1424 w1431] -> w1392
              frame False {
                n312 = Multiply(x=16, y=12) -> (x*y=w1420:i32)
                n313 = for {
                  N: w1420 -> [_]
                  tunnel: ["off"] -> w1424 mode=indexing
                  tunnel: w1417 -> [w1425]
                  tunnel: [w1425] -> w1416
                }
              }
              frame True {
                n314 = for {
                  tunnel: w1448 -> [w1473]
                  tunnel: w1447 -> [w1472]
                  tunnel: w1446 -> [w1471]
                  tunnel: w1445 -> [w1470]
                  tunnel: w1439 -> [w1469]
                  tunnel: string[] ["VPI Test at 23.75V....", "VPI Test at 25.25V....", "VPI Test at 26.75V....", "VPI Test at 28.25V....", "VPI Test at 29.75V....", "VPI Test at 31.25V....", "VPI Test at 32.75V....", "VPI Test at 36.5V....", "VPI Test at 38V....", "VPI Test at 39.5V....", "VPI Test at 41V....", "VPI Test at 42.5V....", "VPI Test at 50V....", "VPI Test at 35V...", "VPI Test at 44V...", "VPI Test at 40.25V..."] -> [w1468] mode=indexing
                  tunnel: w1432 -> [w1467]
                  tunnel: w1433 -> [w1466]
                  tunnel: w1434 -> [w1465]
                  tunnel: [w1464] -> w1440 mode=indexing
                  tunnel: "Bank Cmd" -> [w1463]
                  tunnel: [w1462] -> w1443
                  tunnel: [w1461] -> w1441
                  tunnel: [w1460] -> w1442
                  tunnel: [w1451] -> w1444
                  tunnel: [w1458] -> w1429
                  tunnel: string[] ["074760", "074762", "074764", "074766", "074768", "07476A", "07476C", "074771", "074773", "074775", "074777", "074779", "07477C", "07476F", "07477B", "074776"] -> [w1457] mode=indexing
                  tunnel: "Sequence Names_Test" -> [w1456]
                  tunnel: string[] ["23.75", "25.25", "26.75", "28.25", "29.75", "31.25", "32.75", "36.5", "38", "39.5", "41", "42.5", "50", "35", "44", "40.25"] -> [w1455] mode=indexing
                  i -> [w1459]
                  n315 = Increment(x=w1459) -> (x+1=w1458:i32)
                  n316 = call "WS1050 VPI Test.vi"("Ke2000 Input"=w1472, "AD7747 In"=w1471, "RFFE In"=w1470, "Command"=w1463, "CP Control"=w1457, "error out"=w1473, "Sequence Names"=w1456, "S_ValueC1(pF)"=w1467, "S_ValueC3(pF)"=w1465, "Delay Cap Meas"=w1469, "S_ValueC2(pF)"=w1466, "Status In"=w1468, "VPI Voltage"=w1455) -> ("Data Out"=w1464:string[], "Ke2000 Output"=w1462:refnum<visa-resource-name>, "AD7747 Out"=w1461:refnum<visa-resource-name>, "RFFE Out"=w1460:refnum<visa-resource-name>, "Status"=w1454:string, "IDD_VPI ON"=→"IDD_VPI ON":string, "IDD_VPI OFF"=→"IDD_VPI OFF":string, "error out 2"=w1450:errorcluster)  [unwired: 7 in]
                  n317 = local write "Status"(w1454) -> ()
                  n318 = call "Delay.vi"("error in (no error)"=w1450, "milliseconds to wait"=u32 10) -> ("error out"=w1451:errorcluster)  [unwired: 9 in]
                }
                "VPIData Out" <- w1440
                n319 = Multiply(x=w1429, y=12) -> (x*y=w1428:i32)
                n320 = Reshape Array(w1440, w1428) -> (w1431:string[])
              }
            }
            n321 = Insert Into Array(array=w1400, new element=w1399) -> (w1393:string[])  [unwired: 1 in]
            n322 = Insert Into Array(array=string[] ["074820"], new element=w1387) -> (w1386:string[])  [unwired: 1 in]
            n323 = for {
              tunnel: "CMin Delay" -> [w1415] mode=indexing
              tunnel: [w1414] -> w1391 mode=indexing
              n324 = Decimal String To Number(string=w1415) -> (number=w1414:i32)  [unwired: 2 in, 1 out]
            }
          }
        }
        n325 = flat-sequence {
          tunnel: w707 -> [w890]
          tunnel: w706 -> [w889]
          tunnel: [w888] -> w705
          tunnel: w703 -> [w887]
          tunnel: [w887] -> w702
          frame #0 {
            n326 = Insert Into Array(array=w890, new element=w889) -> (w888:string[])  [unwired: 1 in]
          }
        }
        n327 = case shown="True" w727 {
          tunnel: [w924 w940] -> w788
          tunnel: [w923 w939] -> w787
          tunnel: w730 -> [w926 w938]
          tunnel: w702 -> [w925 w937]
          tunnel: w681 -> [w922 _]
          frame False {
            n328 = for {
              tunnel: w926 -> [w933]
              tunnel: w925 -> [w932]
              tunnel: [w931] -> w924
              tunnel: [w930] -> w923
              tunnel: w922 -> [w927] mode=indexing
              n329 = VISA Write(VISA resource name=w933, write buffer=w927, error in (no error)=w932) -> (VISA resource name out=w930:refnum<visa-resource-name>, error out=w929:errorcluster)  [unwired: 1 out]
              n330 = call "Delay.vi"("error in (no error)"=w929, "milliseconds to wait"=u32 10) -> ("error out"=w931:errorcluster)  [unwired: 9 in]
            }
          }
          frame True {
            n331 = VISA Write(VISA resource name=w938, write buffer="074800", error in (no error)=w937) -> (VISA resource name out=w939:refnum<visa-resource-name>, error out=w936:errorcluster)  [unwired: 1 out]
            n332 = call "Delay.vi"("error in (no error)"=w936, "milliseconds to wait"=u32 10) -> ("error out"=w940:errorcluster)  [unwired: 9 in]
          }
        }
        n333 = case shown="True" w861 {
          tunnel: w788 -> [w950 w976]
          tunnel: w728 -> [w948 w977]
          tunnel: w860 -> [_ w975]
          tunnel: [w950 w972] -> w704
          tunnel: [w947 w964] -> w859
          tunnel: w729 -> [_ w971]
          tunnel: [string[] ["0", "0", "0", "0", "0", "0", "0", "0", "0", "0", "0", "0"] w970] -> w842
          tunnel: [w948 w954] -> w708
          tunnel: w843 -> [_ w965]
          tunnel: w721 -> [w947 w963]
          tunnel: w724 -> [w946 w953]
          tunnel: w723 -> [w945 w952]
          tunnel: w722 -> [w944 w951]
          tunnel: [w946 w953] -> w715
          tunnel: [w945 w952] -> w714
          tunnel: [w944 w951] -> w713
          frame False {
          }
          frame True {
            n334 = local read "Header Table"() -> (w974:string[][])
            n335 = call "WS1050_VSA_AD7747 Updated.vi"("Select Com S0"=w963, "Voltage P1"=w977, "OFFSet Cal"=w953, "Data Record Path"=w971, "Voltage File Path"=w965, "OFFSet Cal 2"=w952, "OFFSet Cal 3"=w951, "error in (no error)"=w976, "Header Table"=w974, "input cluster"=w975) -> ("VSA_V3"=w959:string, "C1_Max(pF)_V1"=w967:string, "VSA_V1"=w966:string, "C2_Max(pF)_V1"=w968:string, "Voltage P1 Out"=w954:refnum<visa-resource-name>, "C3_Max(pF)_V3"=w962:string, "VSA_V 2"=w958:string, "Com Out"=w964:refnum<visa-resource-name>, "C3_Max(pF)_V1"=w969:string, "C1_Max_V2 (pF)"=w957:string, "C1_Max(pF)_V3"=w960:string, "C2_Max(pF)_V3"=w961:string, "C2_Max_V2 (pF)"=w956:string, "C3_Max_V2 (pF)"=w955:string, "error out"=w972:errorcluster)  [unwired: 2 in, 1 out]
            n336 = local write "Status"("Testing VSA....." ("Status")) -> ()
            n337 = Build Array(w966, w967, w968, w969, w958, w957, w956, w955, w959, w960, w961, w962) -> (w970:string[])
          }
        }
        n338 = flat-sequence {
          tunnel: w842 -> [w894]
          tunnel: [w893] -> w841
          tunnel: w705 -> [w892]
          tunnel: w704 -> [w891]
          tunnel: [w891] -> w701
          frame #0 {
            n339 = Insert Into Array(array=w892, new element=w894) -> (w893:string[])  [unwired: 1 in]
          }
        }
        n340 = case shown="True" w716 {
          tunnel: [w1634 w1653] -> w697
          tunnel: w859 -> [w1643 w1659]
          tunnel: [w1643 w1655] -> w808
          tunnel: w701 -> [w1635 w1658]
          tunnel: [w1636 w1656] -> w812
          tunnel: w715 -> [w1642 w1652]
          tunnel: w714 -> [w1641 w1651]
          tunnel: w713 -> [w1640 w1650]
          tunnel: [w1642 w1649] -> w797
          tunnel: [w1641 w1648] -> w796
          tunnel: [w1640 w1647] -> w795
          tunnel: [w1633 w1646] -> w794
          tunnel: w693 -> [w1633 w1646]
          frame False {
            n341 = Multiply(x=4, y=4) -> (x*y=w1639:i32)
            n342 = for {
              N: w1639 -> [_]
              tunnel: ["off"] -> w1636 mode=indexing
              tunnel: w1635 -> [w1644]
              tunnel: [w1644] -> w1634
            }
          }
          frame True {
            n343 = for {
              tunnel: w1658 -> [w1680]
              tunnel: [w1660] -> w1654
              tunnel: w1646 -> [w1679] mode=indexing
              tunnel: w1659 -> [w1678]
              tunnel: [w1674] -> w1657 mode=indexing
              tunnel: [w1667] -> w1655
              tunnel: w1652 -> [w1666]
              tunnel: w1651 -> [w1665]
              tunnel: w1650 -> [w1664]
              tunnel: [w1666] -> w1649
              tunnel: [w1665] -> w1648
              tunnel: [w1664] -> w1647
              n344 = call "Delay.vi"("error in (no error)"=w1680, "milliseconds to wait"=w1679) -> ("error out"=w1675:errorcluster)  [unwired: 9 in]
              n345 = Number To Engineering String(4:w1679) -> (0:w1671:string)  [unwired: 3 in]
              n346 = call "WS1050_AD7747_MeasCAP_Ver1.1.vi"("error in (no error)"=w1675, "OFFSet Cal"=w1666, "AD7747_Number"="8", "Control"=w1678) -> ("error"=w1662:errorcluster, "CAP (pF)"=w1670:string, "Control out"=w1681:refnum<visa-resource-name>)  [unwired: 3 in, 2 out]
              n347 = call "WS1050_AD7747_MeasCAP_Ver1.1.vi"("error in (no error)"=w1662, "OFFSet Cal"=w1665, "AD7747_Number"="9", "Control"=w1681) -> ("error"=w1661:errorcluster, "CAP (pF)"=w1669:string, "Control out"=w1673:refnum<visa-resource-name>)  [unwired: 3 in, 2 out]
              n348 = call "WS1050_AD7747_MeasCAP_Ver1.1.vi"("error in (no error)"=w1661, "OFFSet Cal"=w1664, "AD7747_Number"="a", "Control"=w1673) -> ("error"=w1660:errorcluster, "CAP (pF)"=w1668:string, "Control out"=w1667:refnum<visa-resource-name>)  [unwired: 3 in, 2 out]
              n349 = local write "Status"("Measure Cmin After VSA....." ("Status")) -> ()
              n350 = Build Array(w1671, w1670, w1669, w1668) -> (w1674:string[])
            }
            n351 = call "WS1050_Data Trans.vi"("error in (no error)"=w1654, "Array 2"=w1657) -> ("error out"=w1653:errorcluster, "output array"=w1656:string[])  [unwired: 8 in]
          }
        }
        n352 = local read "Header Table"() -> (w830:string[][])
        n353 = Index Array(array=w830, index (row)=w807, index (col)=2 ("disabled index (col)")) -> (element=w826:string)
        n354 = Index Array(array=w830, index (row)=w807, index (col)=0) -> (element=w832:string)
        n355 = Index Array(array=w830, index (row)=w807, index (col)=1) -> (element=w831:string)
        n356 = flat-sequence {
          tunnel: w841 -> [w886]
          tunnel: [w885] -> w813
          tunnel: w812 -> [w884]
          tunnel: w697 -> [w883]
          tunnel: [w883] -> w685
          frame #0 {
            n357 = Insert Into Array(array=w886, new element=w884) -> (w885:string[])  [unwired: 1 in]
          }
        }
        n358 = Merge Errors(w809, w685) -> (w684:errorcluster)
        n359 = case shown="True" w726 {
          tunnel: w684 -> [w1476 w1520]
          tunnel: w789 -> [w1492 w1559]
          tunnel: [w1492 w1547] -> w810
          tunnel: [w1484 w1536] -> w765
          tunnel: w872 -> [w1491 w1556]
          tunnel: [w1491 w1554] -> w718
          tunnel: w725 -> [_ w1546]
          tunnel: w871 -> [_ w1552]
          tunnel: w808 -> [w1488 w1551]
          tunnel: w793 -> [w1490 w1549]
          tunnel: [w1488 w1531] -> w799
          tunnel: w832 -> [_ w1545]
          tunnel: w831 -> [_ w1544]
          tunnel: w826 -> [_ w1543]
          tunnel: [w1490 w1535] -> w820
          tunnel: [w1486 w1534] -> w815
          tunnel: [w1489 w1532] -> w814
          tunnel: w787 -> [w1487 w1516]
          tunnel: [w1487 w1530] -> w801
          tunnel: w797 -> [_ w1527]
          tunnel: w796 -> [_ w1526]
          tunnel: w795 -> [_ w1525]
          tunnel: w794 -> [_ w1524]
          tunnel: [w1478 w1521] -> w786
          tunnel: "% Amp_T2" -> [_ w1510]
          tunnel: "% Amp_T3" -> [_ w1509]
          tunnel: "% Amp_T1" -> [_ w1511]
          tunnel: [w1474 w1511] -> w676
          tunnel: [w1474 w1510] -> w675
          tunnel: [w1474 w1509] -> w674
          frame False {
            w1474 = 0.0 ("% Amp_T1")
            # "Ke2000"
            n360 = Array Size(array="Driver Name") -> (size(s)=w1481:i32)
            n361 = for {
              N: w1481 -> [_]
              tunnel: "Driver Name" -> [w1496]
              tunnel: [w1498] -> w1479 mode=indexing
              shift-right: [w1493] -> w1475
              shift-left: w1476 -> [w1493]
              i -> [w1494]
              n362 = case shown="1, 3, 18..31, 33, 35, 50..63, 65, 67, 82..95" w1494 {
                tunnel: ["_RT(us)" ("string") "_FT(us)" ("string")] -> w1495
                frame 0, Default {
                }
                frame 1, 3, 18..31, 33, 35, 50..63, 65, 67, 82..95 {
                }
              }
              n363 = Index Array(array=w1496, index=w1494) -> (element=w1502:string)
              n364 = Index Array(array=w1496, index=w1494) -> (element=w1500:string)
              n365 = Concatenate Strings(w1500, "_AMP(v)" ("string")) -> (w1499:string)
              n366 = Concatenate Strings(w1502, w1495) -> (w1497:string)
              n367 = Build Array(w1497, w1499) -> (w1498:string[])
            }
            n368 = Multiply(x=w1481, y=2) -> (x*y=w1477:i32)
            n369 = Reshape Array(w1479, w1477) -> (w1478:string[])
            n370 = for {
              N: w1477 -> [_]
              tunnel: ["off"] -> w1489 mode=indexing
              shift-right: [w1507] -> w1485
              shift-left: w1475 -> [w1507]
            }
            n371 = for {
              N: 16 -> [_]
              tunnel: ["off"] -> w1486 mode=indexing
              shift-right: [w1505] -> w1484
              shift-left: w1485 -> [w1505]
            }
          }
          frame True {
            w1512 = u32 100 ("milliseconds to wait")
            n372 = VISA Close(VISA resource name=w1516, error in (no error)=w1520) -> (error out=w1513:errorcluster)
            n373 = call "Delay.vi"("error in (no error)"=w1513, "milliseconds to wait"=w1512) -> ("error out"=w1514:errorcluster)  [unwired: 9 in]
            n374 = call "Initialize RFFE.vi"("error in (no error)"=w1514, "write buffer"="5", "Select Com Port"=w1516) -> ("error out"=w1519:errorcluster, "VISA resource name out"=w1515:refnum<visa-resource-name>)  [unwired: 7 in]
            n375 = local write "Status"("Switching Time...." ("Status")) -> ()
            n376 = call "Delay.vi"("error in (no error)"=w1519, "milliseconds to wait"=w1512) -> ("error out"=w1517:errorcluster)  [unwired: 9 in]
            n377 = flat-sequence {
              tunnel: [w1581] -> w1558
              tunnel: [w1573] -> w1557
              tunnel: w1556 -> [w1579]
              tunnel: [w1578] -> w1555
              tunnel: w1546 -> [w1577]
              tunnel: w1552 -> [w1576]
              tunnel: [w1570] -> w1550
              tunnel: [w1574] -> w1548
              tunnel: w1545 -> [w1572]
              tunnel: w1544 -> [w1571]
              tunnel: w1517 -> [w1582]
              tunnel: w1559 -> [w1580]
              tunnel: w1551 -> [w1566]
              tunnel: w1549 -> [w1574]
              tunnel: w1543 -> [w1569]
              tunnel: [w1568] -> w1537
              tunnel: w1515 -> [w1567]
              tunnel: [w1566] -> w1528
              tunnel: [w1565] -> w1522
              tunnel: w1510 -> [w1564]
              tunnel: w1511 -> [w1563]
              tunnel: w1509 -> [w1562]
              tunnel: w1558 -> [w1592]
              tunnel: w1557 -> [w1588]
              tunnel: w1555 -> [w1593]
              tunnel: w1550 -> [w1590]
              tunnel: w1548 -> [w1589]
              tunnel: [w1591] -> w1542
              tunnel: [w1593] -> w1541
              tunnel: [w1590] -> w1540
              tunnel: [w1589] -> w1539
              tunnel: [w1588] -> w1538
              tunnel: w1537 -> [w1587]
              tunnel: [w1587] -> w1533
              tunnel: [w1585] -> w1529
              tunnel: w1528 -> [w1585]
              tunnel: [w1583] -> w1523
              tunnel: w1522 -> [w1583]
              tunnel: [w1608] -> w1547
              tunnel: [w1609] -> w1535
              tunnel: [w1610] -> w1554
              tunnel: [w1604] -> w1536
              tunnel: w1542 -> [w1607]
              tunnel: w1541 -> [w1610]
              tunnel: w1540 -> [w1600]
              tunnel: w1539 -> [w1609]
              tunnel: w1538 -> [w1608]
              tunnel: [w1603] -> w1534
              tunnel: w1533 -> [w1602]
              tunnel: [w1602] -> w1532
              tunnel: [w1601] -> w1531
              tunnel: [w1600] -> w1530
              tunnel: w1529 -> [w1599]
              tunnel: w1527 -> [w1598]
              tunnel: w1526 -> [w1597]
              tunnel: w1525 -> [w1596]
              tunnel: w1524 -> [w1595]
              tunnel: w1523 -> [w1594]
              tunnel: [w1594] -> w1521
              frame #0 {
                n378 = call "WS1050_RFFE_ST Scope Single Bit Measurement.vi"("RFFE PIC"=w1567, "A3643A GPIB"=w1580, "% Amp"=w1563, "LOT#"=w1572, "WAFER#"=w1571, "DUT SN"=w1569, "90% Amp"=w1564, "error in (no error)"=w1582, "Scope USB"=w1579, "GROUP"="GROUP", "95% Amp"=w1562, "path"=w1577, "Comment"=w1576) -> ("RFFE PIC 2"=w1570:refnum<visa-resource-name>, "ST Data Out"=w1568:string[], "ST Header Out"=w1565:string[], "Signal"=→"Signal":dbl[], "Scope USB out"=w1578:refnum<visa-resource-name>, "A3643A Out"=w1573:refnum<visa-resource-name>, "Filtered Signal"=→"Filtered Signal":dbl[], "error out"=w1581:errorcluster)  [unwired: 6 in, 1 out]
                "AST" <- w1581
              }
              frame #1 {
                w1586 = u16 0 items=["All Off", "Bank 1", "Bank 2", "Bank 3"] ("Ring")
                n379 = call "WS105x_NI_6501_Relay_Control.vi"("Ring"=w1586, "error in (no error)"=w1592, "Relay_ 10"=FALSE) -> ("error out"=w1591:errorcluster)  [unwired: 3 in, 9 out]
              }
              frame #2 {
                n380 = for {
                  tunnel: w1607 -> [w1630]
                  tunnel: [w1611] -> w1605
                  tunnel: w1595 -> [w1629] mode=indexing
                  tunnel: [w1623] -> w1606 mode=indexing
                  tunnel: w1599 -> [w1621]
                  tunnel: [w1619] -> w1601
                  tunnel: w1598 -> [w1614]
                  tunnel: w1597 -> [w1613]
                  tunnel: w1596 -> [w1612]
                  n381 = call "Delay.vi"("error in (no error)"=w1630, "milliseconds to wait"=w1629) -> ("error out"=w1625:errorcluster)  [unwired: 9 in]
                  n382 = Number To Engineering String(4:w1629) -> (0:w1617:string)  [unwired: 3 in]
                  n383 = call "WS1050_AD7747_MeasCAP_Ver1.1.vi"("error in (no error)"=w1625, "OFFSet Cal"=w1614, "AD7747_Number"="8", "Control"=w1621) -> ("error"=w1631:errorcluster, "CAP (pF)"=w1618:string, "Control out"=w1632:refnum<visa-resource-name>)  [unwired: 3 in, 2 out]
                  n384 = call "WS1050_AD7747_MeasCAP_Ver1.1.vi"("error in (no error)"=w1631, "OFFSet Cal"=w1613, "AD7747_Number"="9", "Control"=w1632) -> ("error"=w1624:errorcluster, "CAP (pF)"=w1616:string, "Control out"=w1622:refnum<visa-resource-name>)  [unwired: 3 in, 2 out]
                  n385 = call "WS1050_AD7747_MeasCAP_Ver1.1.vi"("error in (no error)"=w1624, "OFFSet Cal"=w1612, "AD7747_Number"="a", "Control"=w1622) -> ("error"=w1611:errorcluster, "CAP (pF)"=w1615:string, "Control out"=w1619:refnum<visa-resource-name>)  [unwired: 3 in, 2 out]
                  n386 = local write "Status"("Measure Cmin After ST....." ("Status")) -> ()
                  n387 = Build Array(w1617, w1618, w1616, w1615) -> (w1623:string[])
                }
                n388 = call "WS1050_Data Trans.vi"("error in (no error)"=w1605, "Array 2"=w1606) -> ("error out"=w1604:errorcluster, "output array"=w1603:string[])  [unwired: 8 in]
                "CMin Delay_AST" <- w1603
              }
            }
          }
        }
        n389 = Number To Engineering String(4:w792) -> (0:w834:string)  [unwired: 3 in]
        n390 = Divide(x=w792, y="Delta C Target") -> (x/y=w699:dbl)
        n391 = Multiply(x=w699, y=100.0) -> (x*y=w763:dbl)
        "% Delta Cap" <- w763
        n392 = Number To Engineering String(4:w763) -> (0:w835:string)  [unwired: 3 in]
        n393 = Build Array(w676, w675, w674) -> (w673:dbl[])
        n394 = call "WS1050 EFuse Delta C Setting.vi"("Delta C % Setting"="Delta C % Setting", "error in (no error)"=w765, "Enter DeltaC (pF)"=w763) -> ("error out"=w766:errorcluster, "RFFE Bit Select"=w762:string)  [unwired: 5 in]
        n395 = case shown="True" "BurnIn Efuse" {
          tunnel: w810 -> [w1683 w1690]
          tunnel: w766 -> [w1685 w1696]
          tunnel: [w1683 w1687] -> w711
          tunnel: [w1685 w1699] -> w811
          tunnel: w801 -> [w1684 w1704]
          tunnel: [w1684 w1698] -> w800
          tunnel: [string[] ["n/a", "n/a"] w1697] -> w798
          tunnel: w762 -> [_ w1695]
          frame False {
          }
          frame True {
            # "EFuse Burn-In and Readback Section"
            n396 = VISA Write(VISA resource name=w1704, write buffer=w1695, error in (no error)=w1696) -> (VISA resource name out=w1701:refnum<visa-resource-name>, error out=w1688:errorcluster)  [unwired: 1 out]
            n397 = VISA Write(VISA resource name=w1690, write buffer="VOLT 5.0;;OUTP 1;", error in (no error)=w1688) -> (VISA resource name out=w1687:refnum<visa-resource-name>, error out=w1686:errorcluster)  [unwired: 1 out]
            n398 = call "Delay.vi"("error in (no error)"=w1686, "milliseconds to wait"=u32 100) -> ("error out"=w1702:errorcluster)  [unwired: 9 in]
            n399 = VISA Write(VISA resource name=w1701, write buffer="074901", error in (no error)=w1702) -> (VISA resource name out=w1692:refnum<visa-resource-name>, error out=w1693:errorcluster)  [unwired: 1 out]
            n400 = call "Delay.vi"("error in (no error)"=w1693, "milliseconds to wait"=u32 250) -> ("error out"=w1694:errorcluster)  [unwired: 9 in]
            n401 = case shown="True" TRUE {
              tunnel: [string[] ["n/a", "n/a"] w1717] -> w1697
              tunnel: w1694 -> [w1708 w1725]
              tunnel: [w1708 w1719] -> w1699
              tunnel: w1692 -> [w1706 w1723]
              tunnel: [w1706 w1718] -> w1698
              frame False {
              }
              frame True {
                w1713 = u32 50 ("delay before read (ms)")
                w1712 = "076500" ("write buffer")
                n402 = for {
                  tunnel: w1725 -> [w1731]
                  tunnel: string[] ["074920", "074900"] -> [w1730] mode=indexing
                  tunnel: [w1728] -> w1714
                  tunnel: w1723 -> [w1727]
                  tunnel: [w1726] -> w1711
                  n403 = VISA Write(VISA resource name=w1727, write buffer=w1730, error in (no error)=w1731) -> (VISA resource name out=w1726:refnum<visa-resource-name>, error out=w1728:errorcluster)  [unwired: 1 out]
                  n404 = Wait Until Next ms Multiple(millisecond multiple=u32 100) -> ()  [unwired: 1 out]
                }
                n405 = call "E-Fuse Readback.vi"("write buffer"=w1712, "error in (no error)"=w1714, "delay before read (ms)"=w1713, "VISA resource name"=w1711) -> ("error out"=w1715:errorcluster, "VISA resource name out"=w1716:refnum<visa-resource-name>)  [unwired: 5 in, 1 out]
                n406 = call "E-Fuse Readback.vi"("write buffer"=w1712, "error in (no error)"=w1715, "delay before read (ms)"=w1713, "VISA resource name"=w1716) -> ("error out"=w1721:errorcluster, "EFuse Read Back"=w1709:string, "VISA resource name out"=w1720:refnum<visa-resource-name>)  [unwired: 5 in]
                n407 = call "E-Fuse Readback.vi"("write buffer"=w1712, "error in (no error)"=w1721, "delay before read (ms)"=w1713, "VISA resource name"=w1720) -> ("error out"=w1719:errorcluster, "EFuse Read Back"=w1710:string, "VISA resource name out"=w1718:refnum<visa-resource-name>)  [unwired: 5 in]
                n408 = local write "Status"("EFUSE Read Back R5....." ("Status")) -> ()
                n409 = Build Array(w1709, w1710) -> (w1717:string[])
              }
            }
          }
        }
        "EUSE Burn" <- w798
        n410 = for {
          tunnel: w673 -> [w881] mode=indexing
          tunnel: [w882] -> w672 mode=indexing
          n411 = Multiply(x=w881, y=100.0) -> (x*y=w880:dbl)
          n412 = Number To Fractional String(number=w880) -> (F-format string=w882:string)  [unwired: 3 in]
        }
        n413 = VISA Write(VISA resource name=w800, write buffer="074000", error in (no error)=w811) -> (VISA resource name out=w688:refnum<visa-resource-name>, error out=w824:errorcluster)  [unwired: 1 out]
        n414 = flat-sequence {
          tunnel: [w921] -> w877
          tunnel: [w920] -> w876
          tunnel: [w919] -> w874
          tunnel: w873 -> [w918]
          tunnel: w835 -> [w917]
          tunnel: w834 -> [w916]
          tunnel: [w915] -> w833
          tunnel: w832 -> [w914]
          tunnel: w831 -> [w913]
          tunnel: w828 -> [w912]
          tunnel: w819 -> [w911]
          tunnel: w815 -> [w910]
          tunnel: w814 -> [w909]
          tunnel: w813 -> [w908]
          tunnel: w798 -> [w907]
          tunnel: w786 -> [w906]
          tunnel: w770 -> [w905]
          tunnel: w769 -> [w904]
          tunnel: w729 -> [w902]
          tunnel: w718 -> [w901]
          tunnel: [w901] -> w717
          tunnel: w695 -> [w898]
          tunnel: w694 -> [w897]
          tunnel: w689 -> [w896]
          tunnel: w672 -> [w895]
          frame #0 {
            n415 = local write "Status"("Saving Data....." ("Status")) -> ()
            n416 = call "WS1050_Full Step_RegDump_StepVPI_Ver1.4.vi"("ST Data Out"=w909, "CMin Delay_AST"=w910, "Step Sel"=w904, "% Delta C"=w917, "ST Header Out"=w906, "Efuse Code"="n/a", "error in (no error)"=w911, "VPI_Result"=TRUE, "Lot"=w914, "Wafer"=w913, "Total Delta C"=w916, "TMN DC\\CAP Data Log File Path"=w902, "All Out"=w908, "WS1050 CAP Header"=w905, "Bin File Path"=w918, "% of the Amplitude"=w895, "RB All Regs Dump"=w896, "Test Program"=w912, "EUSE Burn"=w907, "DVA"=w897, "ECAL"=w898) -> ("Pass /Fail?"=w920:bool, "Bins"=w915:string, "Status"=w921:string, "error out"=w919:errorcluster)  [unwired: 2 in, 1 out]
          }
        }
        n417 = call "Delay.vi"("error in (no error)"=w824, "milliseconds to wait"=u32 100) -> ("error out"=w823:errorcluster)  [unwired: 9 in]
        n418 = call "Ke2000 Measurement.vi"("error in (no error)"=w823, "VISA resource name"=w820) -> ("error out"=w819:errorcluster, "Meas in micro"=→"I_stdby End":string, "VISA resource name out"=w806:refnum<visa-resource-name>)  [unwired: 4 in, 3 out]
        n419 = property on="Pass /Fail?" class="Bool (strict)"(error in=w874, "Disabled"=u8 0) -> (error out=w687:errorcluster)  [unwired: 1 in, 1 out]
        n420 = VISA Write(VISA resource name=w711, write buffer="VOLT 0.0", error in (no error)=w687) -> (VISA resource name out=w709:refnum<visa-resource-name>, error out=w712:errorcluster)  [unwired: 1 out]
        n421 = VISA Close(VISA resource name=w688, error in (no error)=w687) -> (error out=→"RFFE Out After Test":errorcluster)
        n422 = local write "Status"(w877) -> ()
        n423 = call "WS105x_NI_6501_Relay_Control.vi"("Ring"=w791, "Relay_ 11"=w790, "error in (no error)"=w712, "Relay_ 10"=w790) -> ("error out"=w720:errorcluster)  [unwired: 2 in, 9 out]
        n424 = flat-sequence {
          tunnel: w720 -> [w943]
          tunnel: [w943] -> w761
          frame #0 {
            n425 = local write "All Out"(string[] []) -> ()
            n426 = One Button Dialog(message="Test Completed") -> ()  [unwired: 1 in, 1 out]
          }
        }
        "Pass /Fail?" <- w876
        "All Out" <- w813
        "Bins" <- w833
        "Completed" <- w761
      }
    }
    "POWER OFF" <- w185
    n427 = case shown="False" w185 {
      tunnel: w156 -> [w495 w503]
      tunnel: [w495 w499] -> w81
      tunnel: w104 -> [w494 w497]
      tunnel: [w494 w496] -> w103
      frame False {
      }
      frame True {
        n428 = call "age364xa Configure Voltage Level.vi"("error in (no error)"=w503, "Level (0.0 Volts)"=0.0, "VISA session"=w497) -> ("error out"=w502:errorcluster, "dup VISA session"=w498:refnum<visa-resource-name>)  [unwired: 7 in]
        n429 = call "age364xa Configure Output Enabled.vi"("error in (no error)"=w502, "Output Enabled (F: Off)"=FALSE, "VISA session"=w498) -> ("error out"=w499:errorcluster, "dup VISA session"=w496:refnum<visa-resource-name>)  [unwired: 7 in]
      }
    }
    "VDD Out Dup" <- w103
    "Power OFF" <- w81
    "Status" <- "Idle....." ("Status")
  }
  n430 = VISA Write(VISA resource name=w11, write buffer="OUTP 0;", error in (no error)=w46) -> (VISA resource name out=w10:refnum<visa-resource-name>, error out=w4:errorcluster)  [unwired: 1 out]
  n431 = call "Ke2400 VI Controler.vi"("ON/OFF"=FALSE, "Voltage Range"=100 ("Voltage Range(V)"), "error in (no error)"=w25, "Current Compliace"=6.0 ("Current Compliance(mA)"), "Volt Level"=0.0 ("Volt Level(V)"), "VISA In"=w26) -> ("error out"=w2:errorcluster, "VISA Out"=→"Ke2400 out":refnum<visa-resource-name>)  [unwired: 4 in]
  n432 = Merge Errors(w4, w3, w2) -> (w1:errorcluster)
  n433 = Build Array(w12, w10, w9, w8, w7) -> (w6:refnum<visa-resource-name>[])
  n434 = for {
    tunnel: w6 -> [w1734] mode=indexing
    shift-right: [w1732] -> w5
    shift-left: w1 -> [w1733]
    n435 = VISA Close(VISA resource name=w1734, error in (no error)=w1733) -> (error out=w1732:errorcluster)
  }
  "Error Out" <- w5
